vi "Main.vi"() -> ()   [LabVIEW 2017]
uses:
  mode_tab.ctl
  state_history.ctl
  <vilib>/Utility/miscctls.llb/LVPointTypeDef.ctl
  <vilib>/Utility/error.llb/DialogType.ctl
  <instrlib>/Gantner Instruments/Ethernet/Gantner-Instruments HighSpeedPort.llb/e.gate Protocol Type.ctl
  global_variable_GAUGE_PANEL_ERROR.vi
  global_variable_STOP.vi
panel:
  out "State History":T1 {"Time Stamp" format="%<%I:%M:%S %p>T"}
  out "STATUS":string
  in  "pause button":bool
  in  "return button":bool
  in  "Mode Tab":T2
  in  "DAQ IP Address":string="192.168.1.28"
  in  "ignore limit switch feedback":bool
  in  "RUN":bool
  in  "debug - run a state":string
  in  "stop program":bool
  in  "set default state":bool
  in  "demo mode":bool
  in  "proceed button":bool
  out "LAST ERROR":errorcluster
  in  "error in (no error)":errorcluster
  out "error out":errorcluster
  # "VIRTUAL CONTROL BOX is still in for loop when program stops connection"
  # "make it easier to add tabs to program"
  # "TAB CONTROL IS NOT RESIZING"
  # "actuation error causes a paused execution (FIXED BY SETTING \"ALLOW DEBUGGING\" TO BE FALSE in vi properties)"
  # "Debug Zone"
  # "The buttons below are now enabled"
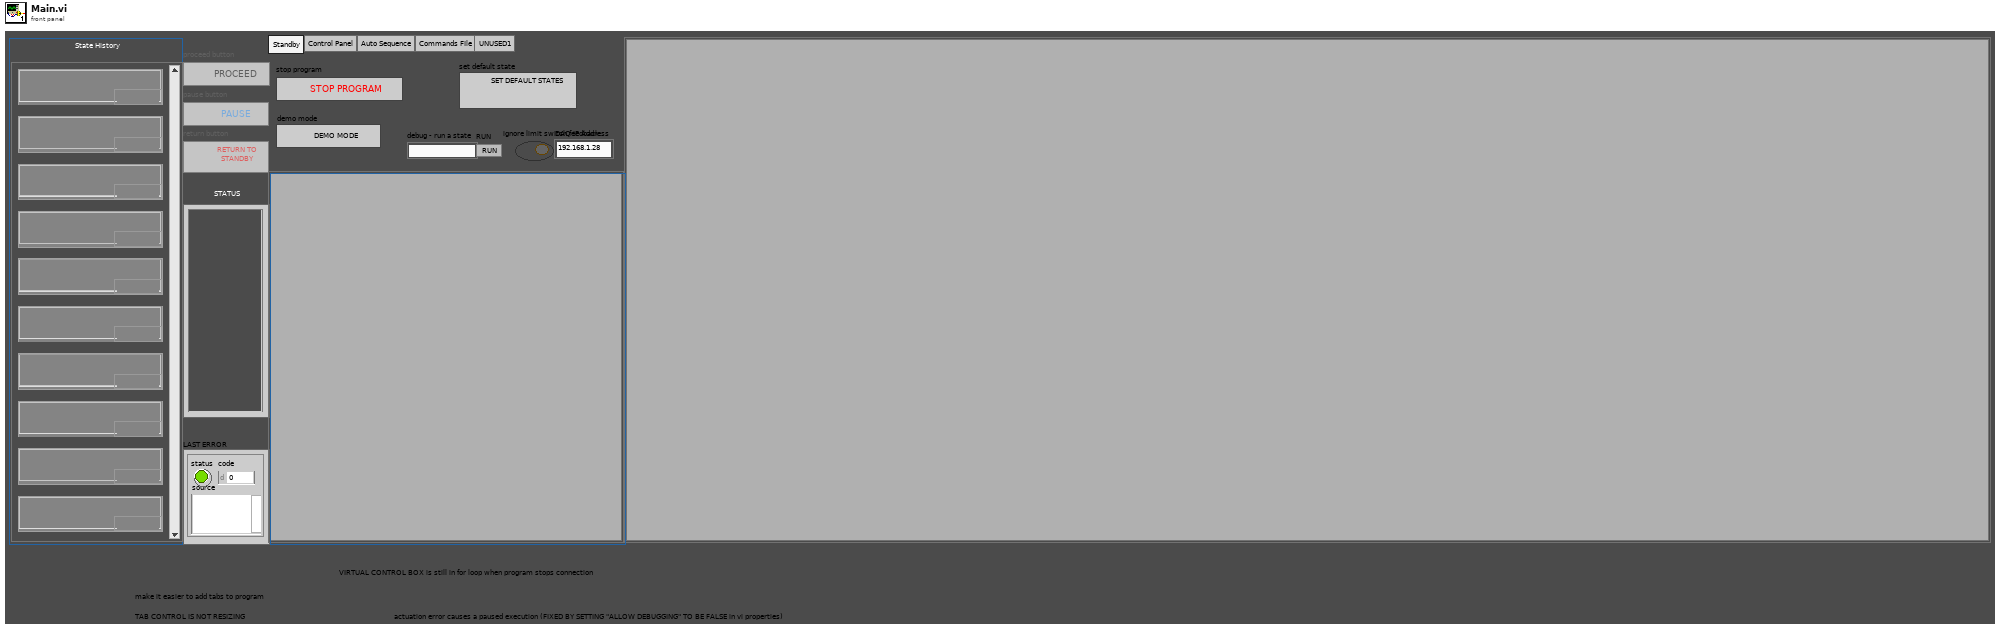
[diagram p1: front panel]
types:
  T1 = typedef "state_history.ctl" = cluster{"String":string, "Time Stamp":timestamp}[]
  T2 = typedef "mode_tab.ctl" = enum32{"Standby", "Control Panel", "Auto Sequence", "Commands FIle", "UNUSED1"}
  T3 = typedef "LVPointTypeDef.ctl" = cluster{"Horizontal":i16, "Vertical":i16}
  T4 = cluster{"name (unnamed)":string, "seconds since 1Jan1904":timestamp}
  T5 = cluster{"name (unnamed)":string, "current time":timestamp}[]
  T6 = enum32{"Invalid", "Standard", "Closed", "Hidden", "Minimized", "Maximized"}
  T7 = enum32{"invalid app kind", "Development System", "Run Time System", "Student Edition", "Embedded LabVIEW", "Evaluation", "Custom"}
  T8 = enum8{"Enabled", "Disabled", "Disabled and Grayed Out"}
  T9 = enum32{"Page Enabled", "Page Disabled", "Page Disabled & Grayed"}
  T10 = enum16{"open/close=1/0", "open/close=0/1", "on/off=1/0", "on/off=0/1"}
  T11 = enum16{"open/close=1/0", "open/close=0/1", "on/off=1/0", "on/off=0/1", "logger_progress"}
  T12 = cluster{"Core":cluster{"Current VI Reference":refnum<vi>, "Close Panel on Exit?":bool}, "time1":dbl, "timeout":dbl, "digital logic":enum16{"open/close=1/0", "open/close=0/1", "on/off=1/0", "on/off=0/1", "logger_progress"}, "channel name":string, "winch parameter":dbl, "proceed button":refnum<vi>, "Mode Tab":refnum<vi>, "mode":enum16{"online", "demo", "compile"}}
  T13 = typedef "DialogType.ctl" = u16
  T14 = cluster{"Current VI Reference":refnum<vi>, "Close Panel on Exit?":bool}
  T15 = typedef "e.gate Protocol Type.ctl" = enum16{"ASCII", "HighspeedPort Online", "HighspeedPort Buffer (giutility.DLL) ", "PostProcessBuffer (giutility.DLL)"}
  T16 = typedef "e.gate Configuration.ctl" = cluster{"connection ID":refnum<k5>, "IPAddress":string, "BufferIndex":i32, "StateMessage":string, "StateCode":i8, "HeaderSize":i32, "BufferSize":i32, "IsBigEndian":i32, "Version":i32, "ChannelCount":i32, "FrameLength":i32, "StartTime":dbl, "dActTimeToSecondFactor":dbl, "StartTimeToDayFactor":dbl, "BufferFillRate":dbl, "SampleRate":dbl, "ChannelData":T17[], "DecodeTimeFormat":string, "SummaryPath":string, "WithCheckSum":i32, "dActTimeDataType":T18, "MaxWriteCount":i32, "MaxReadCount":i32, "TempOffsetRead":i32, "TempLengthRead":i32, "Protocol":T15, "IsSupported":i32, "InputAccessList":i32[], "OutputAccessList":i32[], "DataSource":enum16{"CircleBuffer", "test.con Logger", "test.con Archive"}, "Modules":T19[], "DLL-Handle":T20}
  T17 = typedef "e.gate Channel Data.ctl" = cluster{"VariableName":string, "DataDirection":string, "DataType":string, "DataTypeIndex":T18, "Precision":i16, "FieldLengtht":i16, "ByteCount":i32, "Format":string, "Unit":string, "InputAccessOffset":i32, "OutputAccessOffset":i16, "InputAccessIndex":i16, "OutputAccessIndex":i16, "VarType":string}
  T18 = typedef "e.gate Data Type.ctl" = enum16{"NO", "BOOL", "SINT8", "USINT8", "SINT16", "USINT16", "SINT32", "USINT32", "FLOAT", "SET8", "SET16", "SET32", "DOUBLE", "SINT64", "USINT64", "SET64"}
  T19 = typedef "e.gate Module  Data.ctl" = cluster{"Type":string, "Location":string, "VariablesCount":i16, "UartIndex":i16, "Address":i16, "SystemOffset":i16}
  T20 = typedef "e.gateHSP_DLLhandle.ctl" = cluster{"clientInstance":i32, "connectionInstance":i32, "Is32Bit":bool, "DLL Path":path}
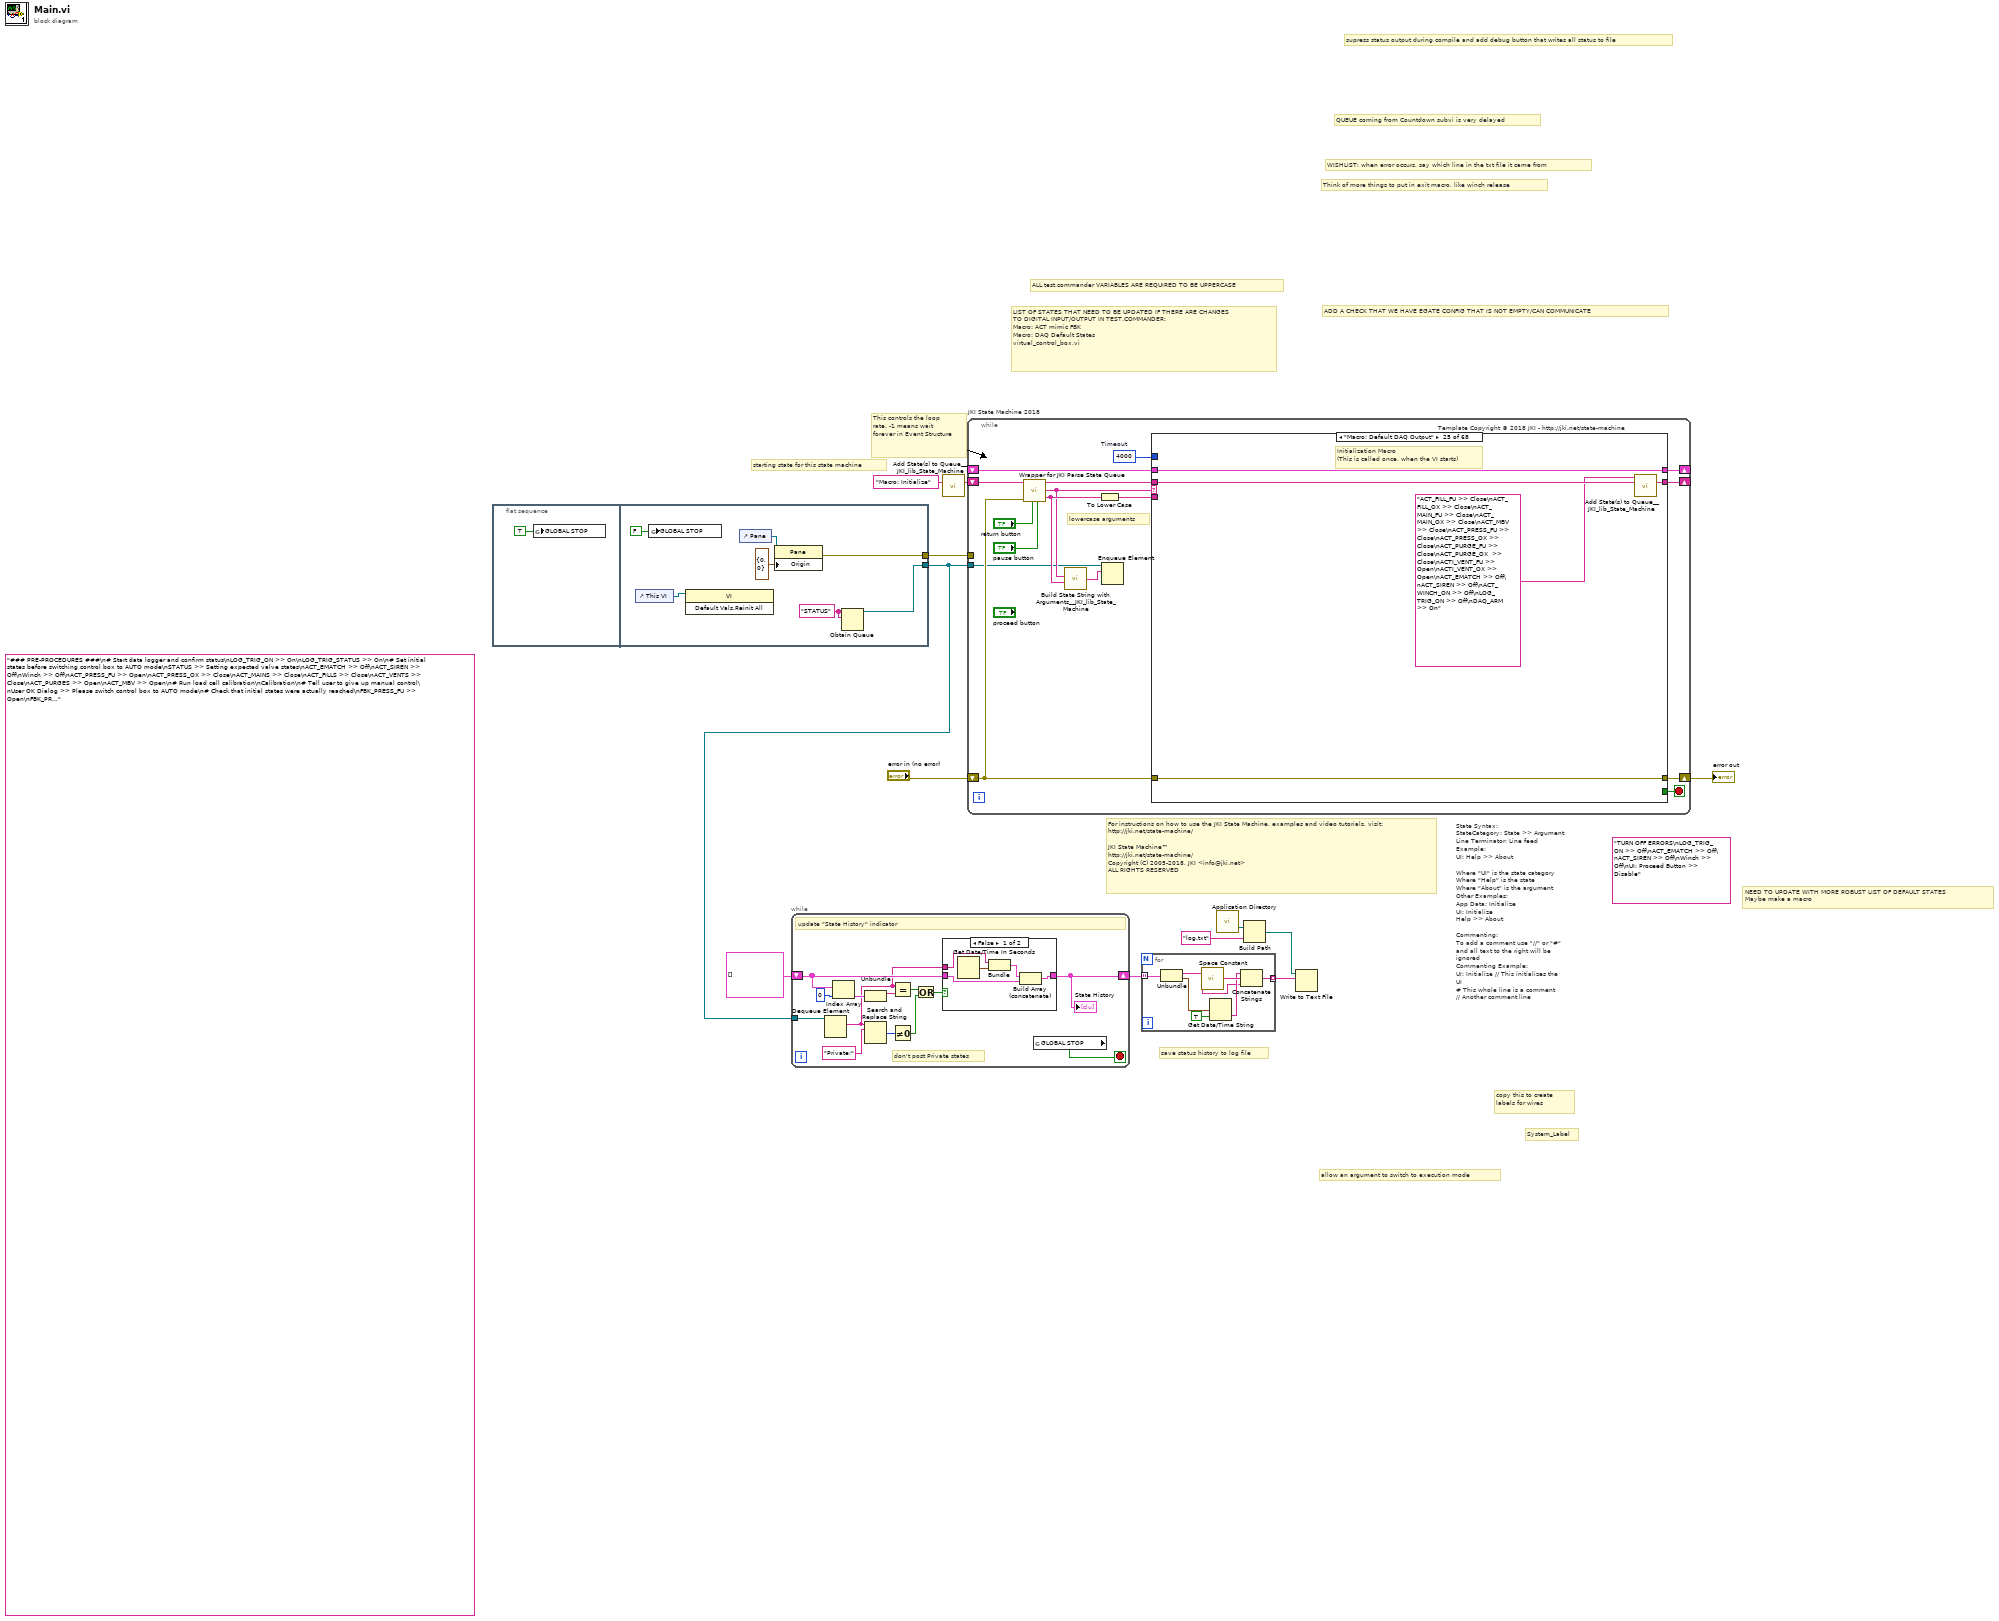
[diagram p0: block diagram]
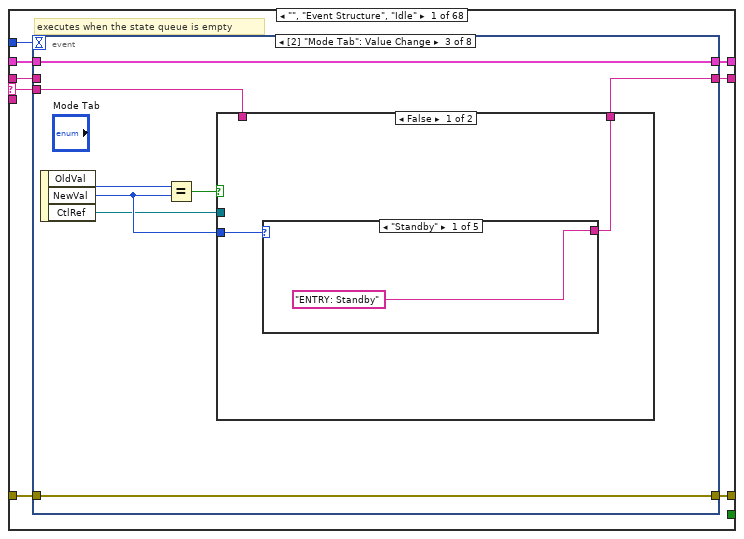
[diagram p3: hidden frame]
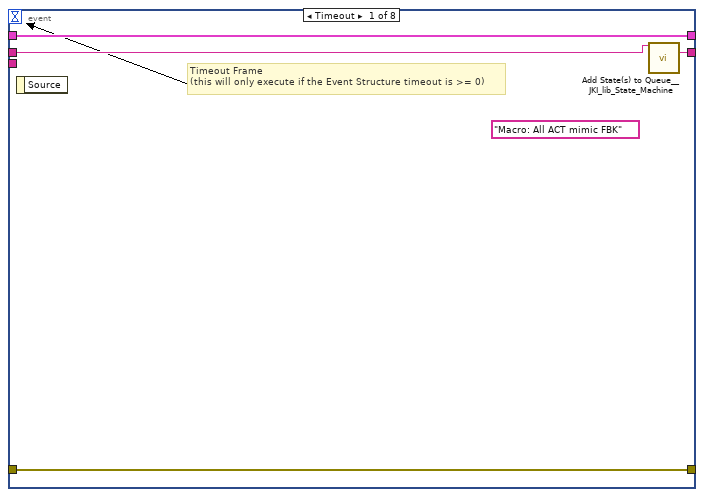
[diagram p4: hidden frame]
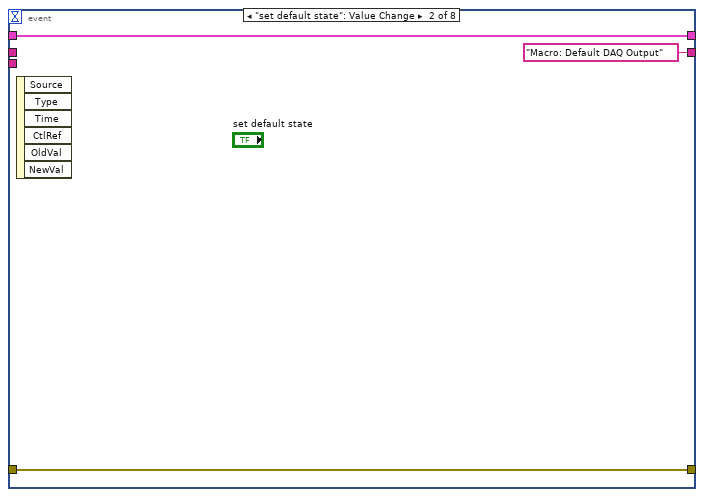
[diagram p5: hidden frame]
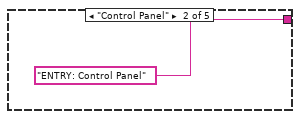
[diagram p6: hidden frame]
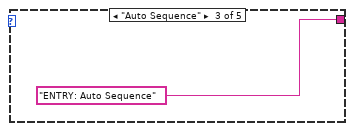
[diagram p7: hidden frame]
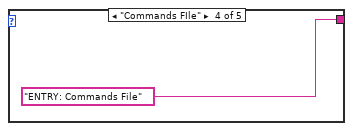
[diagram p8: hidden frame]
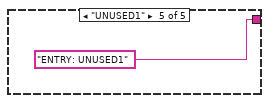
[diagram p9: hidden frame]
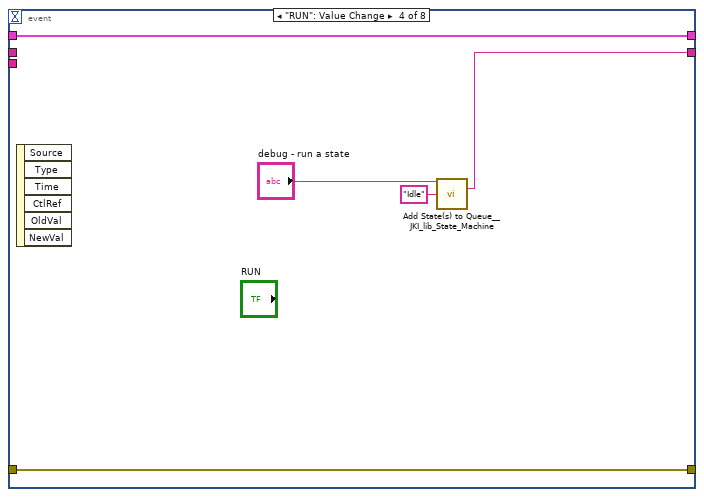
[diagram p11: hidden frame]
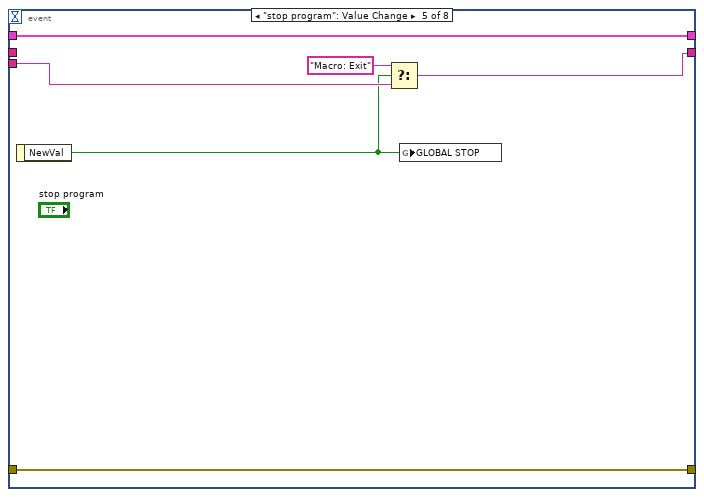
[diagram p12: hidden frame]
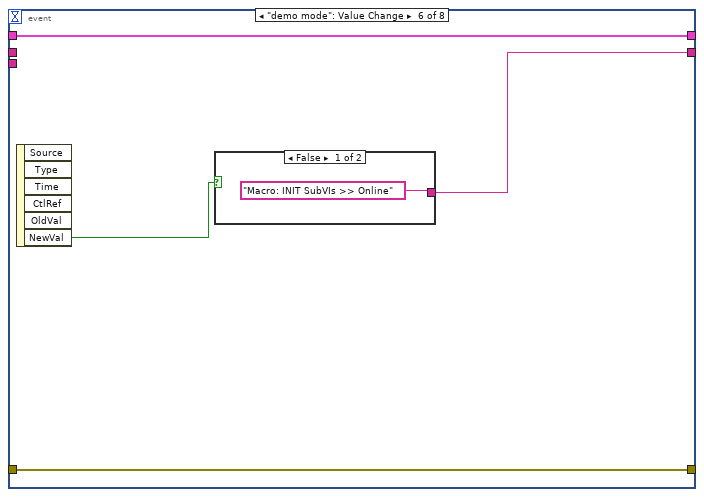
[diagram p13: hidden frame]
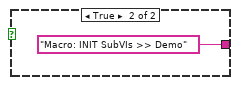
[diagram p14: hidden frame]
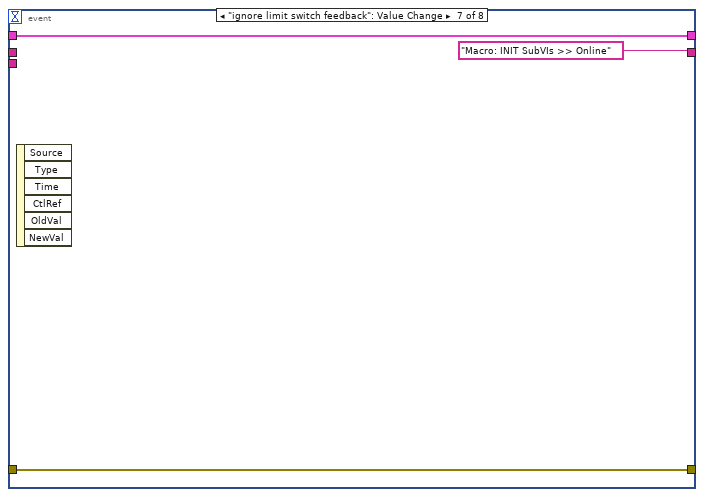
[diagram p15: hidden frame]
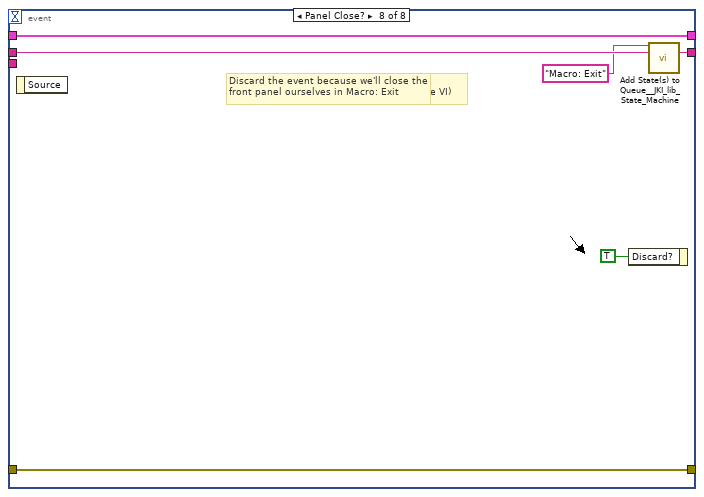
[diagram p16: hidden frame]
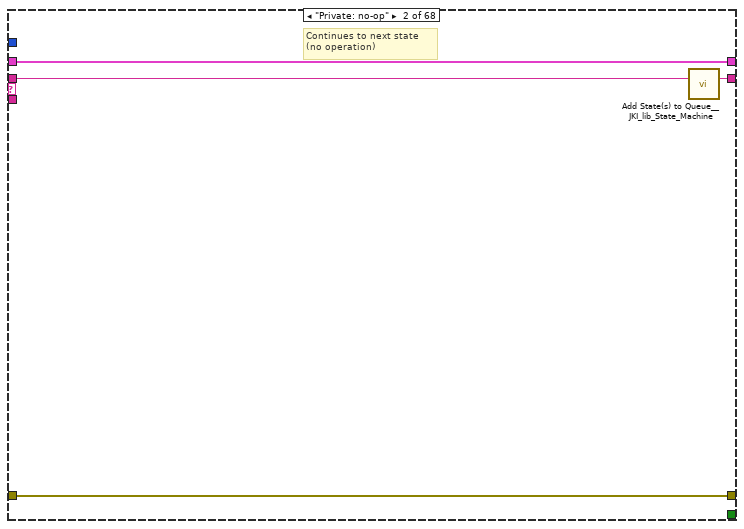
[diagram p17: hidden frame]
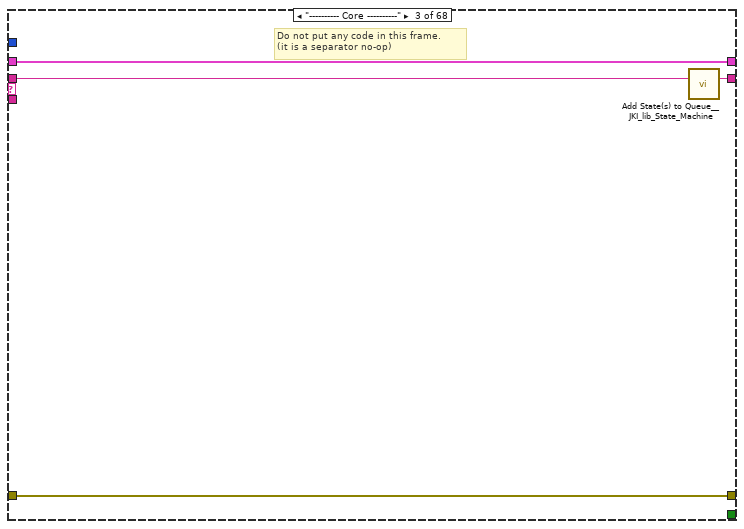
[diagram p18: hidden frame]
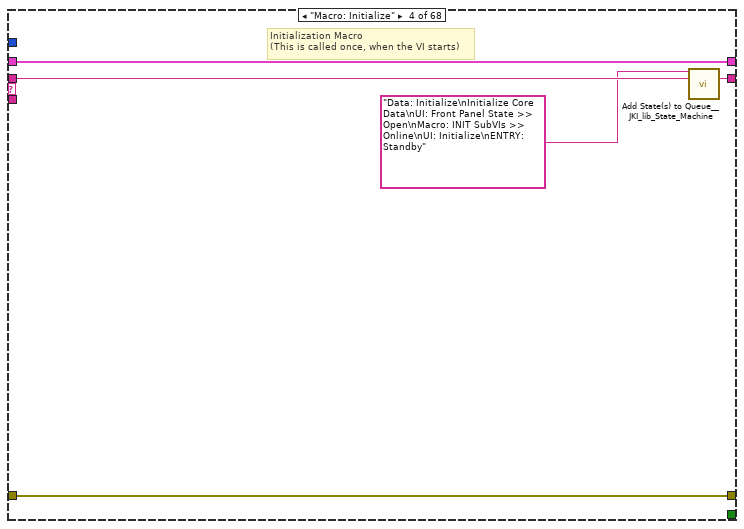
[diagram p19: hidden frame]
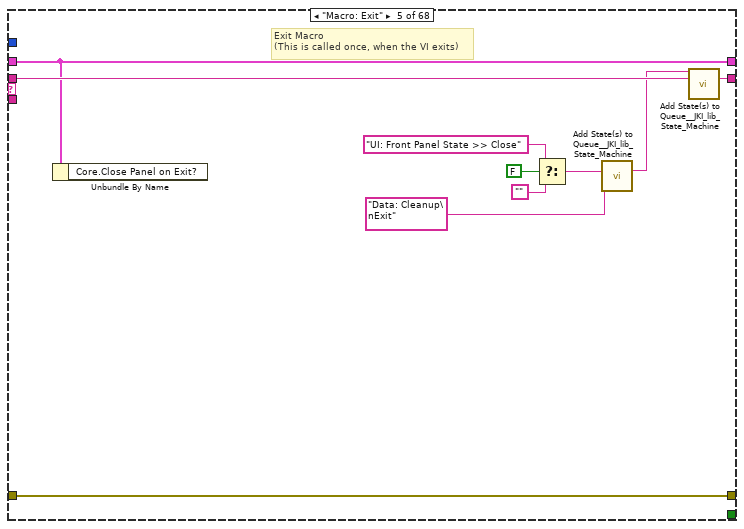
[diagram p20: hidden frame]
diagram:
  (unwired) "TURN OFF ERRORS\nLOG_TRIG_ON >> Off\nACT_EMATCH >> Off\nACT_SIREN >> Off\nWinch >> Off\nUI: Proceed Button >> Disable" ("State(s) in Front (\"\")")
  (unwired) "### PRE-PROCEDURES ###\n# Start data logger and confirm status\nLOG_TRIG_ON >> On\nLOG_TRIG_STATUS >> On\n# Set initial states before switching control box to AUTO mode\nSTATUS >> Setting expected valve states\nACT_EMATCH >> Off\nACT_SIREN >> Off\nWinch >> Off\nACT_PRESS_FU >> Open\nACT_PRESS_OX >> Close\nACT_MAINS >> Close\nACT_FILLS >> Close\nACT_VENTS >> Close\nACT_PURGES >> Open\nACT_MBV >> Open\n# Run load cell calibration\nCalibration\n# Tell user to give up manual control\nUser OK Dialog >> Please switch control box to AUTO mode\n# Check that initial states were actually reached\nFBK_PRESS_FU >> Open\nFBK_PRESS_OX >> Close\nFBK_MAIN_FU >> Close\nFBK_MAIN_OX >> Close\nFBK_FILL_FU >> Close\nFBK_FILL_OX >> Close\nFBK_VENT_FU >> Close\nFBK_VENT_OX >> Close\nFBK_PURGE_FU >> Open\nFBK_PURGE_OX >> Open\nFBK_MBV_OPENED >> Open\n### PROCEDURES ###\n# Begin OX Tank pressurization\nACT_PRESS_OX >> Open\nFBK_PRESS_OX >> Open\nWait for OX Tank Pressure >> 1000 //THE PRESSURE (PSI) THAT THE OX TANK SHOULD REACH\n# Begin countdown procedures\nACT_PURGE_FU >> Close\nACT_PURGE_OX >> Close\nFBK_PURGE_FU >> Close\nFBK_PURGE_OX >> Close\nACT_SIREN >> On\nStart Countdown >> 3 //NUMBER OF SECONDS BETWEEN TURNING ON IGNITION AND OPENING MAIN VALVES\nACT_EMATCH >> On\nACT_SIREN >> Off\nWait >> 3 //NUMBER OF SECONDS BETWEEN TURNING ON IGNITION AND OPENING MAIN VALVES (same as above)\nACT_MAIN_OX >> Open\nWait >> 0.25 //NUMBER OF SECONDS BETWEEN OPENING OX MAIN VALVE AND FU MAIN VALVE\nACT_MAIN_FU >> Open\nFBK_MAIN_OX >> Open\nFBK_MAIN_FU >> Open\n### FIRE ###\nWait >> 0.5 //NUMBER OF SECONDS AFTER THE START OF BURN TO TURN OFF IGNITION (counts towards total burn time)\nACT_EMATCH >> Off\nWait >> 1.5 //NUMBER OF SECONDS AFTER IGNITION TURNS OFF TO OPEN THE PURGES (counts towards total burn time)\nACT_PURGE_FU >> Open\nACT_PURGE_OX >> Open\nWait >> 9 //NUMBER OF SECONDS AFTER PURGES OPEN TO CONTINUE THE BURN (counts towards total burn time)\n### GRACEFUL END ###\nACT_MAIN_OX >> Close\nACT_MAIN_FU >> Close\nFBK_MAIN_OX >> Close\nFBK_MAIN_FU >> Close\nWait >> 4 //NUMBER OF SECONDS TO KEEP PURGES OPEN AFTER MAIN VALVES CLOSED\nACT_PURGE_FU >> Close\nACT_PURGE_OX >> Close\n\n///// probably put the following before purges close ////////\nACT_VENT_FU >> Open\nACT_VENT_OX >> Open\nACT_PRESS_FU >> Close\nACT_PRESS_OX >> Close\nACT_MBV >> Close\n//////  ///////\n\nFBK_MBV_CLOSED >> Close\n\n//////// still need to do this?? ////////\nACT_PRESS_FU >> Open\nFBK_PRESS_OX >> Open\nWait >> 2\nACT_PRESS_FU >> Close\nACT_PRESS_OX >> Close\n//////  ///////\n\n### FINISH ###\nLOG_TRIG_ON >> Off\nWait >> 30\n###Ask to run cleanup?"
  # "save status history to log file"
  # "ALL test.commander VARIABLES ARE REQUIRED TO BE UPPERCASE"
  # "LIST OF STATES THAT NEED TO BE UPDATED IF THERE ARE CHANGES\nTO DIGITAL INPUT/OUTPUT IN TEST.COMMANDER:\nMacro: ACT mimic FBK\nMacro: DAQ Default States\nvirtual_control_box.vi"
  # "allow an argument to switch to execution mode"
  # "supress status output during compile and add debug button that writes all status to file"
  # "NEED TO UPDATE WITH MORE ROBUST LIST OF DEFAULT STATES\nMaybe make a macro"
  # "QUEUE coming from Countdown subvi is very delayed"
  # "WISHLIST: when error occurs, say which line in the txt file it came from"
  # "starting state for this state machine"
  # "Think of more things to put in exit macro, like winch release"
  # "ADD A CHECK THAT WE HAVE EGATE CONFIG THAT IS NOT EMPTY/CAN COMMUNICATE"
  # "For instructions on how to use the JKI State Machine, examples and video tutorials, visit:\nhttp://jki.net/state-machine/\n\nJKI State Machine™\nhttp://jki.net/state-machine/\nCopyright (C) 2005-2018, JKI <info@jki.net>\nALL RIGHTS RESERVED"
  # "State Syntax:\nStateCategory: State >> Argument\nLine Terminator: Line feed\nExample:\nUI: Help >> About\n\nWhere \"UI\" is the state category\nWhere \"Help\" is the state\nWhere \"About\" is the argument\nOther Examples:\nApp Data: Initialize\nUI: Initialize\nHelp >> About\n\nCommenting:\nTo add a comment use \"//\" or \"#\" and all text to the right will be ignored\nCommenting Example:\nUI: Initialize // This initializes the UI\n# This whole line is a comment\n// Another comment line"
  # "copy this to create labels for wires"
  # "This controls the loop rate. -1 means wait forever in Event Structure"
  # "System_Label"
  n1 = flat-sequence {
    tunnel: [w17] -> w6
    tunnel: [w14] -> w4
    frame #0 {
      n2 = global write "global_variable_STOP.vi" "GLOBAL STOP"(TRUE ("GLOBAL STOP")) -> ()
    }
    frame #1 {
      w15 = "STATUS" ("name (unnamed)")
      n3 = control-ref of="This VI"() -> (w20:refnum<vi>)
      n4 = global write "global_variable_STOP.vi" "GLOBAL STOP"(FALSE ("GLOBAL STOP")) -> ()
      n5 = invoke class="VI" method="Default Vals.Reinit All"(reference=w20) -> ()  [unwired: 2 in, 3 out]
      n6 = control-ref of="Pane"() -> (w18:refnum<vi>)
      n7 = property class="Pane"(reference=w18, "Origin"=T3 {"Horizontal"=0, "Vertical"=0}) -> (error out=w17:errorcluster)  [unwired: 1 in, 1 out]
      n8 = Obtain Queue(name (unnamed)=w15, element data type=w15) -> (queue out=w14:refnum<queue>)  [unwired: 3 in, 2 out]
    }
  }
  n9 = while {
    shift-right: [w21] -> w9
    shift-left: cluster{string, "current time":timestamp}[] [] -> [w31]
    tunnel: w4 -> [w22]
    stop <- w23 stop-if-true
    # "don't post Private states"
    # "update \"State History\" indicator"
    n10 = Dequeue Element(queue=w22) -> (element=w27:string)  [unwired: 2 in, 3 out]
    n11 = Index Array(array=w31, index=0) -> (element=w32:cluster{string, "current time":timestamp})
    n12 = Unbundle(w32) -> (w30:string)  [unwired: 1 out]
    n13 = Search and Replace String(input string=w27, search string="Private:") -> (number of replacements=w26:i32)  [unwired: 6 in, 3 out]
    n14 = Equal?(x=w27, y=w30) -> (x = y?=w29:bool)
    n15 = Not Equal To 0?(x=w26) -> (x != 0?=w24:bool)
    n16 = Or(x=w29, y=w24) -> (x .or. y?=w25:bool)
    n17 = case shown="False" w25 {
      tunnel: [w38 w39] -> w21
      tunnel: w27 -> [w37 _]
      tunnel: w31 -> [w35 w39]
      frame False {
        n18 = Get Date/Time In Seconds() -> (seconds since 1Jan1904=w34:timestamp)
        n19 = Bundle("name (unnamed)"=w37, "seconds since 1Jan1904"=w34) -> (w36:T4)  [unwired: 1 in]
        n20 = Build Array (concatenate)(w36, w35) -> (w38:T5)
      }
      frame True {
      }
    }
    "State History" <- w21
    n21 = global read "global_variable_STOP.vi" "GLOBAL STOP"() -> (w23:bool)
  }
  n22 = call <vilib>:"Add State(s) to Queue__JKI_lib_State_Machine.vi"("State(s) in (\"\")"="Macro: Initialize") -> ("States Out"=w12:string)  [unwired: 14 in]
  n23 = while "JKI State Machine 2018" {
    shift-right: [w52] -> _
    shift-left: _ -> [w51]
    shift-right: [w55] -> w5
    shift-left: "error in (no error)" -> [w47]
    shift-right: [w54] -> _
    shift-left: w12 -> [w46]
    tunnel: w6 -> [_]
    tunnel: w4 -> [w41]
    stop <- w53 stop-if-true
    w50 = 4000  # Timeout
    # "lowercase arguments"
    # "Template Copyright © 2018 JKI - http://jki.net/state-machine"
    n24 = call "Wrapper for JKI Parse State Queue.vi"("pause execution"="pause button", "cancel execution"="return button", "error in (no error)"=w47, "State Queue"=w46) -> ("Arguments"=w43:string, "Current State"=w42:string, "Remaining States"=w48:string)  [unwired: 5 in]
    n25 = call <vilib>:"Build State String with Arguments__JKI_lib_State_Machine.vi"("Arguments (\"\")"=w43, "State"=w42) -> ("State with Arguments"=w40:string)  [unwired: 4 in]
    n26 = To Lower Case(string=w43) -> (all lower case string=w49:string)
    n27 = Enqueue Element(queue=w41, element=w40) -> ()  [unwired: 2 in, 3 out]
    n28 = case shown="\"Macro: Default DAQ Output\"" w42 {
      selector: w42 -> [w56 _ _ _ _ w136 _ _ _ _ _ _ _ _ _ _ _ _ _ _ _ _ _ _ _ _ _ _ _ _ _ _ _ _ _ _ _ _ w690 w732 w762 _ _ _ _ w837 w849 _ w941 w982 _ _ _ _ _ w1058 w1068 w1078 _ w1114 w1186 w1203 w1220 w1237 _ _ _ _]
      tunnel: w48 -> [w63 w116 w120 w125 w135 w140 w159 w166 w222 w226 w239 w245 w249 w254 w260 w271 w345 w368 w378 w391 w404 w414 w424 w430 w435 w437 w443 w459 w477 w492 w497 w513 w519 w525 w538 w625 w627 w634 w675 w734 w763 w768 w790 w795 w801 w834 w846 w885 w904 w945 w987 w1002 w1006 w1010 w1011 w1067 w1077 w1087 w1091 w1119 w1188 w1205 w1222 w1239 w1250 w1256 w1261 w1264]
      tunnel: w49 -> [_ _ _ _ _ _ _ _ _ _ _ _ _ _ w255 w265 w343 w362 w372 w387 w401 w409 _ _ _ _ _ w448 _ _ _ w512 _ _ w553 _ _ w646 w689 w725 w748 w767 _ w791 w803 w836 w848 w870 w916 w963 w989 _ _ _ w1015 w1063 w1073 w1083 _ w1111 w1183 w1200 w1217 w1234 _ _ _ w1263]
      tunnel: w51 -> [w61 w113 w117 w122 w132 w138 w152 w163 w220 w223 _ w240 w246 w250 w258 w267 w340 w365 w375 w385 w400 w411 w421 w425 w432 w439 w445 w457 w481 w494 w509 w514 w521 w536 w552 w622 w628 w633 w673 w735 w747 w765 w787 w792 w806 w825 w844 w883 w932 w976 w986 w999 w1003 w1007 w1017 w1061 w1071 w1081 w1088 w1105 w1193 w1210 w1227 w1244 w1247 w1251 w1258 w1275]
      tunnel: [w60 w114 w118 w123 w133 w142 w156 w165 w219 w224 w236 w241 w247 w252 w256 w268 w341 w366 w376 w383 w402 w412 w422 w428 w433 w440 w446 w455 w478 w495 w498 w511 w522 w526 w540 w623 w629 w642 w682 w730 w759 w769 w788 w793 w810 w833 w845 w886 w939 w980 w988 w1000 w1004 w1008 w1019 w1065 w1075 w1085 w1089 w1116 w1194 w1211 w1228 w1245 w1248 w1254 w1259 w1266] -> w55
      tunnel: w47 -> [w59 w114 w118 w123 w133 w141 w156 w167 w219 w224 w236 w242 w247 w252 w257 w269 w342 w366 w376 w384 w402 w412 w422 w428 w433 w440 w446 w456 w478 w495 w499 w511 w522 w527 w550 w623 w629 w644 w687 w731 w761 w770 w788 w793 w809 w833 w845 w860 w939 w980 w988 w1000 w1004 w1008 w1018 w1065 w1075 w1085 w1089 w1110 w1194 w1211 w1228 w1245 w1248 w1254 w1259 w1267]
      tunnel: [w62 w115 w119 w124 w134 w139 w158 w170 w221 w225 w238 w244 w248 w253 w259 w270 w344 w367 w377 w390 w403 w413 w423 w429 w434 w441 w447 w458 w482 w496 w510 w515 w523 w537 w559 w624 w630 w657 w696 w736 w764 w771 w789 w794 w813 w840 w852 w887 w942 w983 w990 w1001 w1005 w1009 w1020 w1066 w1076 w1086 w1090 w1118 w1195 w1212 w1229 w1246 w1249 w1255 w1260 w1276] -> w54
      tunnel: [_ _ _ _ _ _ _ w164 TRUE _ _ _ _ _ _ _ _ _ _ _ _ _ _ _ _ _ _ _ _ _ _ _ _ _ _ _ _ _ _ _ _ _ _ _ _ _ _ _ _ _ _ _ _ _ _ _ _ _ _ _ _ _ _ _ _ _ _ _] -> w53
      tunnel: [w58 w113 w117 w122 w132 w138 w157 w163 w220 w223 w237 w240 w246 w250 w258 w267 w340 w365 w375 w385 w400 w411 w421 w425 w432 w439 w445 w457 w481 w494 w509 w514 w521 w536 w551 w622 w628 w640 w672 w735 w747 w765 w787 w792 w804 w825 w844 w881 w932 w976 w986 w999 w1003 w1007 w1017 w1060 w1070 w1080 w1088 w1105 w1192 w1209 w1226 w1243 w1247 w1251 w1258 w1275] -> w52
      tunnel: w50 -> [w57 _ _ _ _ _ _ _ _ _ _ _ _ _ _ _ _ _ _ _ _ _ _ _ _ _ _ _ _ _ _ _ _ _ _ _ _ _ _ _ _ _ _ _ _ _ _ _ _ _ _ _ _ _ _ _ _ _ _ _ _ _ _ _ _ _ _ _]
      frame "", "Event Structure", "Idle" {
        # "executes when the state queue is empty"
        n29 = event shown="[2] \"Mode Tab\": Value Change" {
          selector: _ -> [_ _ _ _ _ _ _ _]
          dyn-events: _ -> [_ _ _ _ _ _ _ _]
          timeout: w57 -> [_ _ _ _ _ _ _ _]
          tunnel: w63 -> [w64 _ _ _ _ _ _ w112]
          tunnel: [w67 "Macro: Default DAQ Output" ("States Out") w73 w87 w95 w101 "Macro: INIT SubVIs >> Online" ("States Out") w111] -> w62
          tunnel: w61 -> [w65 w68 w76 w91 w94 w98 w104 w109]
          tunnel: [w66 w69 w75 w90 w93 w99 w105 w110] -> w60
          tunnel: w59 -> [w66 w69 w75 w90 w93 w99 w105 w110]
          tunnel: [w65 w68 w76 w91 w94 w98 w104 w109] -> w58
          tunnel: w56 -> [_ _ w72 _ w97 _ _ _]
          event Timeout {
            (unwired) "Macro: All ACT mimic FBK" ("State(s) in Front (\"\")")
            # "Timeout Frame\n(this will only execute if the Event Structure timeout is >= 0)"
            n30 = event-data() -> ()  [unwired: 1 in, 1 out]
            n31 = call <vilib>:"Add State(s) to Queue__JKI_lib_State_Machine.vi"("State(s) in Front (\"\")"=w64) -> ("States Out"=w67:string)  [unwired: 14 in]
          }
          event "set default state": Value Change {
            n32 = event-data() -> ()  [unwired: 1 in, 6 out]
          }
          event Value Change {
            n33 = event-data() -> ("OldVal"=w77:T2, "NewVal"=w74:T2, "CtlRef"=w71:refnum<vi>)  [unwired: 1 in]
            n34 = Equal?(x=w77, y=w74) -> (x = y?=w78:bool)
            n35 = case shown="False" w78 {
              tunnel: [w79 w86] -> w73
              tunnel: w74 -> [w80 _]
              tunnel: w72 -> [_ w86]
              tunnel: w71 -> [_ _]
              frame False {
                n36 = case shown="\"Standby\"" w80 {
                  tunnel: ["ENTRY: Standby" "ENTRY: Control Panel" "ENTRY: Auto Sequence" ("string") "ENTRY: Commands File" "ENTRY: UNUSED1"] -> w79
                  frame "Standby" {
                  }
                  frame "Control Panel" {
                  }
                  frame "Auto Sequence" {
                  }
                  frame "Commands FIle" {
                  }
                  frame "UNUSED1" {
                  }
                }
              }
              frame True {
              }
            }
          }
          event "RUN": Value Change {
            n37 = event-data() -> ()  [unwired: 1 in, 6 out]
            n38 = call <vilib>:"Add State(s) to Queue__JKI_lib_State_Machine.vi"("State(s) in Front (\"\")"="debug - run a state", "State(s) at Back (\"\")"="Idle" ("State(s) at Back (\"\")")) -> ("States Out"=w87:string)  [unwired: 13 in]
          }
          event "stop program": Value Change {
            n39 = event-data() -> ("NewVal"=w92:bool)  [unwired: 1 in]
            n40 = Select(t="Macro: Exit", s=w92, f=w97) -> (s? t:f=w95:string)
            n41 = global write "global_variable_STOP.vi" "GLOBAL STOP"(w92) -> ()
          }
          event "demo mode": Value Change {
            n42 = event-data() -> ("NewVal"=w100:bool)  [unwired: 1 in, 5 out]
            n43 = case shown="False" w100 {
              tunnel: ["Macro: INIT SubVIs >> Online" ("States Out") "Macro: INIT SubVIs >> Demo" ("States Out")] -> w101
              frame False {
              }
              frame True {
              }
            }
          }
          event "ignore limit switch feedback": Value Change {
            n44 = event-data() -> ()  [unwired: 1 in, 6 out]
          }
          event Panel Close? {
            # "Discard the event because we'll close the front panel ourselves in Macro: Exit"
            # "Close Panel button (pressed) Event\n(this executes Macro: Exit to terminate the VI)"
            n45 = event-data() -> ()  [unwired: 1 in, 1 out]
            n46 = event-data("Discard?"=TRUE) -> ()  [unwired: 1 in, 1 out]
            n47 = call <vilib>:"Add State(s) to Queue__JKI_lib_State_Machine.vi"("State(s) in Front (\"\")"="Macro: Exit", "State(s) in (\"\")"=w112) -> ("States Out"=w111:string)  [unwired: 13 in]
          }
        }
      }
      frame "Private: no-op" {
        # "Continues to next state\n(no operation)"
        n48 = call <vilib>:"Add State(s) to Queue__JKI_lib_State_Machine.vi"("State(s) in (\"\")"=w116) -> ("States Out"=w115:string)  [unwired: 14 in]
      }
      frame "---------- Core ----------" {
        # "Do not put any code in this frame.\n(it is a separator no-op)"
        n49 = call <vilib>:"Add State(s) to Queue__JKI_lib_State_Machine.vi"("State(s) in (\"\")"=w120) -> ("States Out"=w119:string)  [unwired: 14 in]
      }
      frame "Macro: Initialize" {
        # "Initialization Macro\n(This is called once, when the VI starts)"
        n50 = call <vilib>:"Add State(s) to Queue__JKI_lib_State_Machine.vi"("State(s) in Front (\"\")"="Data: Initialize\nInitialize Core Data\nUI: Front Panel State >> Open\nMacro: INIT SubVIs >> Online\nUI: Initialize\nENTRY: Standby", "State(s) in (\"\")"=w125) -> ("States Out"=w124:string)  [unwired: 13 in]
      }
      frame "Macro: Exit" {
        # "Exit Macro\n(This is called once, when the VI exits)"
        n51 = Unbundle By Name(w132) -> ()  [unwired: 1 out]
        n52 = Select(t="UI: Front Panel State >> Close", s=FALSE, f="") -> (s? t:f=w129:string)
        n53 = call <vilib>:"Add State(s) to Queue__JKI_lib_State_Machine.vi"("State(s) in (\"\")"=w129, "State(s) at Back (\"\")"="Data: Cleanup\nExit") -> ("States Out"=w127:string)  [unwired: 13 in]
        n54 = call <vilib>:"Add State(s) to Queue__JKI_lib_State_Machine.vi"("State(s) in Front (\"\")"=w127, "State(s) in (\"\")"=w135) -> ("States Out"=w134:string)  [unwired: 13 in]
      }
      frame Default {
        w145 = 42 items=["No error", "Argument error", "Memory is full", "Out of zone", "End of file", "File already open", "Generic file I/O error", "File not found", "File permission error", "Disk is full", "Duplicate path", "Too many files open", "System feature not enabled", "Resource file not found", "Cannot add resource", "Resource not found", "Image not found", "Image memory error", "Pen does not exist", "Config type invalid", "Config token not found", "Config parse error", "Config memory error", "Bad external code format", "Bad external code offset", "External code not present", "Null window", "Destroy window error", "Null menu", "Print aborted", "Bad print record", "Print driver error", "Windows error during printing", "Memory error during printing", "Print dialog error", "Generic print error", "Invalid device refnum", "Device not found", "Device parameter error", "Device unit error", "Cannot open device", "Device call aborted", "Generic error", "Cancelled by user", "Object ID too low", "Object ID too high", "Object not in heap", "Unknown heap", "Unknown object (invalid DefProc)", "Unknown object (DefProc not in table)", "Message out of range", "Invalid (null) method", "Unknown message", "Manager call not supported", "Bad address", "Network operation in progress", "Network operation timed out", "Connection is busy", "Network attribute not supported", "Network error", "Address in use", "System out of memory", "Connection aborted", "Connection refused", "Not connected", "Already connected", "Connection closed", "Initialization error (interapplication manager)", "Bad occurrence", "Wait on unbound occurrence handler", "Occurrence queue overflow", "Datalog type conflict", "Unused", "Unrecognized type (interapplication manager)", "Memory corrupt", "Failed to make temporary DLL", "Old CIN version", "Drag socket not found", "Failed to load drop-object", "Failed to register OLE object", "Failed to release OLE object", "Format specifier type mismatch", "Unknown format specifier", "Too few format specifiers", "Too many format specifiers", "Scan failed", "Newer CIN version", "Error converting to variant", "Runtime menu error", "Password tampered", "Variant attribute not found", "Incompatible variant data type", "Event data is not available", "Event Store is not present", "Occurrence is not found", "Event Queue is not created", "Event info is not available", "Refnum passed is NULL", "Error retrieving Class GUID", "Error retrieving CoClass GUID", "Error retrieving TypeLib GUID.", "Bad built application magic bytes.", "Specific driver is different from the specific driver associated with the Logical Name.", "There is no session opened to the class driver.", "Max Error", "MAX - Error with config objects", "MAX - Error loading configuration", "MAX - Group not supported"]
        # "Current State"
        # "Do not delete, rename, or modify this frame.\n(this is used to capture unhandled states and typos)"
        # "Handle mistyped state name (developer tool)"
        n55 = Format Into String(format string="Software Exception: Unhandled State \"%s\"." ("message"), error in=w141, w136) -> (resulting string=w144:string, error out=w143:errorcluster)  [unwired: 1 in]
        n56 = call <vilib>:"Error Cluster From Error Code.vi"("show call chain? (False)"=TRUE, "error in (no error)"=w143, "error message (\"\")"=w144, "error code (0)"=w145) -> ("error out"=w142:errorcluster)  [unwired: 5 in]
        n57 = call <vilib>:"Add State(s) to Queue__JKI_lib_State_Machine.vi"("State(s) in (\"\")"=w140) -> ("States Out"=w139:string)  [unwired: 14 in]
      }
      frame "Initialize Core Data" {
        # "Do not delete, rename, or modify this frame.\n(this is used to determine panel behavior on exit)"
        # "originally closed?"
        # "exe?"
        # "If panel starts closed or is an EXE, then close it when we exit"
        n58 = property class="VI"() -> ("FP.State"=w149:T6)  [unwired: 2 in, 2 out]
        n59 = property class="App"() -> ("App.Kind"=w155:T7)  [unwired: 2 in, 2 out]
        n60 = control-ref of="Current VI Reference"() -> (w150:refnum<vi>)
        n61 = Equal?(x=w149, y=T6."Standard" ("Front Panel Window:State")) -> (x = y?=w147:bool)
        n62 = Equal?(x=w155, y=T7."Run Time System" ("Application:Kind")) -> (x = y?=w153:bool)
        n63 = Or(x=w147, y=w153) -> (x .or. y?=w151:bool)
        n64 = Bundle By Name(cluster=w152, "Core.Current VI Reference"=w150, "Core.Close Panel on Exit?"=w151) -> (w157:T12)
        n65 = call <vilib>:"Add State(s) to Queue__JKI_lib_State_Machine.vi"("State(s) in (\"\")"=w159) -> ("States Out"=w158:string)  [unwired: 14 in]
      }
      frame "Error Handler" {
        # "Handle any errors here.\nYou can also output any states to clean-up after errors occur"
        n66 = Unbundle By Name(w167) -> ("code"=w161:i32, "source"=w169:string)
        n67 = Unbundle By Name(w163) -> ("mode"=w162:enum16{"online", "demo", "compile"})
        n68 = case shown="Default" w162 {
          tunnel: w169 -> [w177 w199]
          tunnel: [w176 w198] -> w168
          tunnel: w167 -> [w175 w197]
          tunnel: w166 -> [_ w196]
          tunnel: [w173 w195] -> w165
          tunnel: [w172 w194] -> w164
          tunnel: w161 -> [w171 w192]
          tunnel: [w174 w193] -> w160
          frame "compile" {
            # "In this mode if we get a generic error it's probably a bad state from\nAUTO_SEQUENCE_COMMANDS.txt"
            n69 = case shown="66" w171 {
              tunnel: w177 -> [w178 w188 _]
              tunnel: [w178 "Macro: INIT SubVIs >> Online\nENTRY: Standby" "Macro: INIT SubVIs >> Online\nENTRY: Standby"] -> w176
              tunnel: w175 -> [w180 w184 w190]
              tunnel: [w182 w184 w190] -> w174
              tunnel: [w181 w185 w189] -> w173
              tunnel: [w179 _ _] -> w172
              frame Default {
                w179 = TRUE ("GLOBAL STOP")
                w183 = T13 2 items=["no dialog", "OK message", "continue or stop message", "OK message + warnings", "continue/stop + warnings"] ("type of dialog (OK msg:1)")
                n70 = global write "global_variable_STOP.vi" "GLOBAL STOP"(w179) -> ()
                n71 = call <vilib>:"General Error Handler.vi"("type of dialog (OK msg:1)"=w183, "error in (no error)"=w180) -> ("error out"=w182:errorcluster)  [unwired: 9 in, 4 out]
                n72 = call <vilib>:"Clear Errors.vi"("error in (no error)"=w180) -> ("error out"=w181:errorcluster)  [unwired: 5 in, 1 out]
              }
              frame 42 {
                # "generic error, unhandled state"
                n73 = One Button Dialog(message=w188, button name ("OK")="Return to Standby" ("T button name (\"OK\")")) -> ()  [unwired: 1 out]
                n74 = call <vilib>:"Clear Errors.vi"("error in (no error)"=w184) -> ("error out"=w185:errorcluster)  [unwired: 5 in, 1 out]
              }
              frame 66 {
                # "lost qstation connection"
                n75 = call <vilib>:"Clear Errors.vi"("error in (no error)"=w190) -> ("error out"=w189:errorcluster)  [unwired: 5 in, 1 out]
              }
            }
          }
          frame Default {
            n76 = case shown="66" w192 {
              tunnel: w199 -> [_ w212 _]
              tunnel: [w204 w209 "Macro: INIT SubVIs >> Online\nENTRY: Standby"] -> w198
              tunnel: w197 -> [w202 w206 w215]
              tunnel: w196 -> [w204 w208 _]
              tunnel: [w203 w207 w217] -> w195
              tunnel: [w201 _ _] -> w194
              tunnel: [w200 w206 w215] -> w193
              frame Default {
                w201 = TRUE ("GLOBAL STOP")
                w205 = T13 2 items=["no dialog", "OK message", "continue or stop message", "OK message + warnings", "continue/stop + warnings"] ("type of dialog (OK msg:1)")
                n77 = global write "global_variable_STOP.vi" "GLOBAL STOP"(w201) -> ()
                n78 = call <vilib>:"General Error Handler.vi"("type of dialog (OK msg:1)"=w205, "error in (no error)"=w202) -> ("error out"=w200:errorcluster)  [unwired: 9 in, 4 out]
                n79 = call <vilib>:"Clear Errors.vi"("error in (no error)"=w202) -> ("error out"=w203:errorcluster)  [unwired: 5 in, 1 out]
              }
              frame 108 {
                n80 = call <vilib>:"Clear Errors.vi"("error in (no error)"=w206) -> ("error out"=w207:errorcluster)  [unwired: 5 in, 1 out]
                n81 = Two Button Dialog(message=w212, 1:"Proceed Anyway (NOT RECOMMENDED)" ("F button name (\"Cancel\")"), 2:"Return to Standby" ("T button name (\"OK\")")) -> (T button?=w210:bool)
                n82 = Select(t="ENTRY: Standby", s=w210, f=w208) -> (s? t:f=w209:string)
              }
              frame 66 {
                # "lost qstation connection"
                n83 = call <vilib>:"Clear Errors.vi"("error in (no error)"=w215) -> ("error out"=w217:errorcluster)  [unwired: 5 in, 1 out]
              }
            }
          }
        }
        "LAST ERROR" <- w160
        n84 = call <vilib>:"Add State(s) to Queue__JKI_lib_State_Machine.vi"("State(s) in Front (\"\")"=w168) -> ("States Out"=w170:string)  [unwired: 14 in]
      }
      frame "Exit" {
        # "Do not put any code in this frame.\n(No errors that occur here will be handled.)"
        n85 = call <vilib>:"Add State(s) to Queue__JKI_lib_State_Machine.vi"("State(s) in (\"\")"=w222) -> ("States Out"=w221:string)  [unwired: 14 in]
      }
      frame "---------- Data ----------" {
        # "Do not put any code in this frame.\n(It is a separator no-op. You can make a copy of this frame to create a new Data frame)"
        n86 = call <vilib>:"Add State(s) to Queue__JKI_lib_State_Machine.vi"("State(s) in (\"\")"=w226) -> ("States Out"=w225:string)  [unwired: 14 in]
      }
      frame "Data: Initialize" {
        w228 = enum16{"online", "demo", "compile"}."online"  # mode
        w230 = 0.0  # winch parameter
        w231 = ""  # channel name
        w232 = T11."open/close=1/0"  # digital logic
        w233 = 0.0  # timeout
        w234 = 0.0  # time1
        w235 = T14 {"Current VI Reference"=refnum, "Close Panel on Exit?"=FALSE}  # Core
        # "do not delete - used by framework"
        # "Expand Bundle to add new data elements to shift register data."
        # "Data names and types of shift register data are defined by this bundle."
        # "Initialize the shift-register data, here.\n(data names are defined by what you wire into the bundle function)"
        n87 = control-ref of="proceed button"() -> (w229:refnum<vi>)
        n88 = control-ref of="Mode Tab"() -> (w227:refnum<vi>)
        n89 = Bundle("Core"=w235, "time1"=w234, "timeout"=w233, "digital logic"=w232, "channel name"=w231, "winch parameter"=w230, "proceed button"=w229, "Mode Tab"=w227, "mode"=w228) -> (w237:T12)  [unwired: 1 in]
        n90 = call <vilib>:"Add State(s) to Queue__JKI_lib_State_Machine.vi"("State(s) in (\"\")"=w239) -> ("States Out"=w238:string)  [unwired: 14 in]
      }
      frame "Data: Cleanup" {
        # "Cleanup any data and references, here.\n(this is called automatically, by the Macro: Exit)"
        n91 = Unbundle By Name(w240) -> ("Core.Current VI Reference"=w243:refnum<vi>)
        n92 = Close Reference(reference=w243, error in (no error)=w242) -> (error out=w241:errorcluster)
        n93 = call <vilib>:"Add State(s) to Queue__JKI_lib_State_Machine.vi"("State(s) in (\"\")"=w245) -> ("States Out"=w244:string)  [unwired: 14 in]
      }
      frame "---------- UI ----------" {
        # "Do not put any code in this frame.\n(It is a separator no-op. You can make a copy of this frame to create a new UI frame)"
        n94 = call <vilib>:"Add State(s) to Queue__JKI_lib_State_Machine.vi"("State(s) in (\"\")"=w249) -> ("States Out"=w248:string)  [unwired: 14 in]
      }
      frame "UI: Initialize" {
        # "Initialize the User Interface, here.\n(this is called automatically, by the Macro: Init)"
        n95 = call <vilib>:"Add State(s) to Queue__JKI_lib_State_Machine.vi"("State(s) in Front (\"\")"="UI: All Tabs >> Disable\nPrivate: Gauge Panel\nPrivate: Control Panel", "State(s) in (\"\")"=w254) -> ("States Out"=w253:string)  [unwired: 13 in]
      }
      frame "UI: Cursor Set" {
        # "Argument"
        # "Set and Unset Cursor Busy.\n(Usage: \"UI: Cursor Set >> Busy|Idle\")"
        n96 = case shown="\"idle\", Default" w255 {
          tunnel: w257 -> [w262 w264]
          tunnel: [w261 w263] -> w256
          frame "idle", Default {
            n97 = call <vilib>:"Unset Busy.vi"("error in (no error)"=w262) -> ("error out"=w261:errorcluster)  [unwired: 10 in]
          }
          frame "busy" {
            n98 = call <vilib>:"Set Busy.vi"("error in (no error)"=w264) -> ("error out"=w263:errorcluster)  [unwired: 9 in, 1 out]
          }
        }
        n99 = call <vilib>:"Add State(s) to Queue__JKI_lib_State_Machine.vi"("State(s) in (\"\")"=w260) -> ("States Out"=w259:string)  [unwired: 14 in]
      }
      frame "UI: Front Panel State" {
        # "Argument"
        # "Set Front Panel Open or Closed\n(Usage: \"UI: Front Panel State >> Open|Close\")"
        n100 = Unbundle By Name(w267) -> ("Core.Current VI Reference"=w266:refnum<vi>)
        n101 = case shown="\"open\", \"standard\", Default" w265 {
          tunnel: w269 -> [w277 w292 w303 w316 w329]
          tunnel: [w279 w293 w305 w318 w331] -> w268
          tunnel: w266 -> [w278 w290 w304 w317 w330]
          frame "open", "standard", Default {
            w272 = T6."Standard" ("State")
            n102 = property class="VI"(reference=w278, error in=w277) -> (reference out=w275:refnum<vi>, error out=w276:errorcluster, "FP.State"=w274:T6)
            n103 = Not Equal?(x=w274, y=w272) -> (x != y?=w273:bool)
            n104 = case shown="True" w273 {
              tunnel: [w283 w285] -> w279
              tunnel: w276 -> [w282 w285]
              tunnel: w275 -> [w281 _]
              tunnel: w272 -> [w280 _]
              frame True {
                n105 = invoke class="VI" method="FP.Open"(reference=w281, error in=w282, "Activate"=TRUE, "State"=w280) -> (error out=w283:errorcluster)  [unwired: 1 in, 4 out]
              }
              frame False {
              }
            }
          }
          frame "close", "closed" {
            n106 = property class="VI"(reference=w290, error in=w292) -> (reference out=w289:refnum<vi>, error out=w291:errorcluster, "FP.State"=w287:T6)
            n107 = Not Equal?(x=w287, y=T6."Closed" ("Front Panel Window:State")) -> (x != y?=w286:bool)
            n108 = case shown="True" w286 {
              tunnel: [w294 w297] -> w293
              tunnel: w291 -> [w294 w296]
              tunnel: w289 -> [_ w295]
              frame False {
              }
              frame True {
                n109 = invoke class="VI" method="FP.Close"(reference=w295, error in=w296) -> (error out=w297:errorcluster)  [unwired: 1 in, 2 out]
              }
            }
          }
          frame "hidden", "hide" {
            w298 = T6."Hidden" ("State")
            n110 = property class="VI"(reference=w304, error in=w303) -> (reference out=w301:refnum<vi>, error out=w302:errorcluster, "FP.State"=w300:T6)
            n111 = Not Equal?(x=w300, y=w298) -> (x != y?=w299:bool)
            n112 = case shown="True" w299 {
              tunnel: [w309 w310] -> w305
              tunnel: w302 -> [w308 w310]
              tunnel: w301 -> [w307 _]
              tunnel: w298 -> [w306 _]
              frame True {
                n113 = invoke class="VI" method="FP.Open"(reference=w307, error in=w308, "State"=w306) -> (error out=w309:errorcluster)  [unwired: 2 in, 4 out]
              }
              frame False {
              }
            }
          }
          frame "minimize", "minimized" {
            w311 = T6."Minimized" ("State")
            n114 = property class="VI"(reference=w317, error in=w316) -> (reference out=w314:refnum<vi>, error out=w315:errorcluster, "FP.State"=w313:T6)
            n115 = Not Equal?(x=w313, y=w311) -> (x != y?=w312:bool)
            n116 = case shown="True" w312 {
              tunnel: [w322 w323] -> w318
              tunnel: w315 -> [w321 w323]
              tunnel: w314 -> [w320 _]
              tunnel: w311 -> [w319 _]
              frame True {
                n117 = invoke class="VI" method="FP.Open"(reference=w320, error in=w321, "State"=w319) -> (error out=w322:errorcluster)  [unwired: 2 in, 4 out]
              }
              frame False {
              }
            }
          }
          frame "maximize", "maximized" {
            w324 = T6."Maximized" ("State")
            n118 = property class="VI"(reference=w330, error in=w329) -> (reference out=w327:refnum<vi>, error out=w328:errorcluster, "FP.State"=w326:T6)
            n119 = Not Equal?(x=w326, y=w324) -> (x != y?=w325:bool)
            n120 = case shown="True" w325 {
              tunnel: [w335 w336] -> w331
              tunnel: w328 -> [w334 w336]
              tunnel: w327 -> [w333 _]
              tunnel: w324 -> [w332 _]
              frame True {
                n121 = invoke class="VI" method="FP.Open"(reference=w333, error in=w334, "State"=w332) -> (error out=w335:errorcluster)  [unwired: 2 in, 4 out]
              }
              frame False {
              }
            }
          }
        }
        n122 = call <vilib>:"Add State(s) to Queue__JKI_lib_State_Machine.vi"("State(s) in (\"\")"=w271) -> ("States Out"=w270:string)  [unwired: 14 in]
      }
      frame "UI: Proceed Button" {
        # "Enable/Disable the \"Proceed\" UI button\n(the button value affects \"Wait...\" states)"
        n123 = Unbundle By Name(w340) -> ("proceed button"=w339:refnum<vi>, "mode"=w338:enum16{"online", "demo", "compile"})
        n124 = case shown="\"online\", \"demo\", Default" w338 {
          tunnel: [TRUE ("Blinking") FALSE ("Blinking")] -> w337
          frame "compile" {
          }
          frame "online", "demo", Default {
          }
        }
        n125 = case shown="\"disable\"" w343 {
          tunnel: w339 -> [w351 w357]
          tunnel: w342 -> [w350 w359]
          tunnel: [w349 w358] -> w341
          tunnel: w337 -> [w348 w354]
          frame "disable" {
            n126 = property class="Bool (strict)"(reference=w351, error in=w350, "Blinking"=FALSE ("Value"), "DisabledEnum"=T8."Disabled and Grayed Out" ("Disabled"), "Value"=w348) -> (error out=w349:errorcluster)  [unwired: 1 out]
          }
          frame "enable", Default {
            n127 = property class="Bool (strict)"(reference=w357, error in=w359, "Blinking"=TRUE ("Value"), "DisabledEnum"=T8."Enabled" ("Disabled"), "Value"=w354) -> (error out=w358:errorcluster)  [unwired: 1 out]
          }
        }
        n128 = call <vilib>:"Add State(s) to Queue__JKI_lib_State_Machine.vi"("State(s) in (\"\")"=w345) -> ("States Out"=w344:string)  [unwired: 14 in]
      }
      frame "UI: Pause Button" {
        # "Wait until Proceed Button is hit, then start auto sequence\n(This is called from \"Idle\" state)"
        n129 = case shown="\"disable\"" w362 {
          tunnel: [T8."Disabled and Grayed Out" ("Disabled") T8."Enabled" ("Disabled")] -> w361
          frame "disable" {
          }
          frame "enable", Default {
          }
        }
        n130 = control-ref of="pause button"() -> (w363:refnum<vi>)
        n131 = property class="Bool (strict)"(reference=w363, "DisabledEnum"=w361, "Value"=FALSE) -> ()  [unwired: 1 in, 2 out]
        n132 = Wait (ms)(milliseconds to wait=u32 50) -> ()  [unwired: 1 out]
        n133 = call <vilib>:"Add State(s) to Queue__JKI_lib_State_Machine.vi"("State(s) in (\"\")"=w368) -> ("States Out"=w367:string)  [unwired: 14 in]
      }
      frame "UI: Return Button" {
        # "Wait until Proceed Button is hit, then start auto sequence\n(This is called from \"Idle\" state)"
        n134 = case shown="\"enable\", Default" w372 {
          tunnel: [T8."Disabled and Grayed Out" ("Disabled") T8."Enabled" ("Disabled")] -> w371
          frame "disable" {
          }
          frame "enable", Default {
          }
        }
        n135 = control-ref of="return button"() -> (w373:refnum<vi>)
        n136 = property class="Bool"(reference=w373, "DisabledEnum"=w371) -> ()  [unwired: 1 in, 2 out]
        n137 = Wait (ms)(milliseconds to wait=u32 50) -> ()  [unwired: 1 out]
        n138 = call <vilib>:"Add State(s) to Queue__JKI_lib_State_Machine.vi"("State(s) in (\"\")"=w378) -> ("States Out"=w377:string)  [unwired: 14 in]
      }
      frame "UI: One Tab Enable" {
        # "Enables the tab passed as an argument\n(zero-indexed, from left to right)"
        n139 = Unbundle By Name(w385) -> ("Mode Tab"=w381:refnum<vi>)
        n140 = Decimal String To Number(string=w387) -> (number=w386:i32)  [unwired: 2 in, 1 out]
        n141 = property class="TabCtl (strict)"(reference=w381, error in=w384, "DisabledEnum"=T8."Enabled" ("Disabled")) -> (error out=w383:errorcluster, "Pages"=w388:refnum<vi>[])  [unwired: 1 out]
        n142 = for {
          tunnel: w388 -> [w395] mode=indexing
          tunnel: w386 -> [w393]
          i -> [w394]
          # "one tab"
          n143 = Equal?(x=w393, y=w394) -> (x = y?=w392:bool)
          n144 = case shown="True" w392 {
            tunnel: w395 -> [_ w397]
            frame False {
            }
            frame True {
              n145 = property class="Page"(reference=w397, "PageEnb"=T9."Page Enabled" ("Page Enabled State")) -> ()  [unwired: 1 in, 2 out]
            }
          }
        }
        n146 = Wait (ms)(milliseconds to wait=u32 50) -> ()  [unwired: 1 out]
        n147 = call <vilib>:"Add State(s) to Queue__JKI_lib_State_Machine.vi"("State(s) in (\"\")"=w391) -> ("States Out"=w390:string)  [unwired: 14 in]
      }
      frame "UI: Change Tabs" {
        # "Sets the active tab based on the argument passed\n(zero-indexed, from left to right)"
        n148 = Decimal String To Number(string=w401) -> (number=w399:i32)  [unwired: 2 in, 1 out]
        n149 = Unbundle By Name(w400) -> ("Mode Tab"=w398:refnum<vi>)
        n150 = property class="TabCtl (strict)"(reference=w398, "Value"=w399) -> ()  [unwired: 1 in, 2 out]
        n151 = call <vilib>:"Add State(s) to Queue__JKI_lib_State_Machine.vi"("State(s) in (\"\")"=w404) -> ("States Out"=w403:string)  [unwired: 14 in]
      }
      frame "UI: All Tabs" {
        # "Wait until Proceed Button is hit, then start auto sequence\n(This is called from \"Idle\" state)"
        n152 = case shown="\"enable\", Default" w409 {
          tunnel: [T9."Page Disabled & Grayed" ("Page Enabled State") T9."Page Enabled" ("Page Enabled State")] -> w408
          tunnel: [T8."Disabled and Grayed Out" ("Disabled") T8."Enabled" ("Disabled")] -> w406
          frame "disable" {
          }
          frame "enable", Default {
          }
        }
        n153 = control-ref of="Mode Tab"() -> (w405:refnum<vi>)
        n154 = property class="TabCtl (strict)"(reference=w405, "DisabledEnum"=w406) -> ("Pages"=w407:refnum<vi>[])  [unwired: 1 in, 2 out]
        n155 = for {
          tunnel: w408 -> [w416]
          tunnel: w407 -> [w415] mode=indexing
          # "all tabs"
          n156 = property class="Page"(reference=w415, "PageEnb"=w416) -> ()  [unwired: 1 in, 2 out]
        }
        n157 = Wait (ms)(milliseconds to wait=u32 50) -> ()  [unwired: 1 out]
        n158 = call <vilib>:"Add State(s) to Queue__JKI_lib_State_Machine.vi"("State(s) in (\"\")"=w414) -> ("States Out"=w413:string)  [unwired: 14 in]
      }
      frame "---------- Macro ----------" {
        # "Do not put any code in this frame.\n(It is a separator no-op. You can make a copy of this frame to create a new Macro frame)"
        n159 = call <vilib>:"Add State(s) to Queue__JKI_lib_State_Machine.vi"("State(s) in (\"\")"=w424) -> ("States Out"=w423:string)  [unwired: 14 in]
      }
      frame "ENTRY: Standby" {
        # "Set up UI and prepare to enter \"Standby\" tab"
        n160 = Wait (ms)(milliseconds to wait=u32 50) -> ()  [unwired: 1 out]
        n161 = call <vilib>:"Add State(s) to Queue__JKI_lib_State_Machine.vi"("State(s) in Front (\"\")"="STATUS >> Standby\nACT_EMATCH >> Off\nACT_SIREN >> Off\nPrivate: Winch action >> Off\nUI: Return Button >> Disable\nUI: Pause Button >> Disable\nUI: Proceed Button >> Disable\nUI: All Tabs >> Enable\nUI: Change Tabs >> 0\nPrivate: Sub Panel Control Panel >> Disable\nIdle", "State(s) in (\"\")"=w430) -> ("States Out"=w429:string)  [unwired: 13 in]
      }
      frame "Macro: Default DAQ Output" {
        # "Initialization Macro\n(This is called once, when the VI starts)"
        n162 = call <vilib>:"Add State(s) to Queue__JKI_lib_State_Machine.vi"("State(s) in Front (\"\")"="ACT_FILL_FU >> Close\nACT_FILL_OX >> Close\nACT_MAIN_FU >> Close\nACT_MAIN_OX >> Close\nACT_MBV >> Close\nACT_PRESS_FU >> Close\nACT_PRESS_OX >> Close\nACT_PURGE_FU >> Close\nACT_PURGE_OX  >> Close\nACTI_VENT_FU >> Open\nACTI_VENT_OX >> Open\nACT_EMATCH >> Off\nACT_SIREN >> Off\nACT_WINCH_ON >> Off\nLOG_TRIG_ON >> Off\nDAQ_ARM >> On", "State(s) in (\"\")"=w435) -> ("States Out"=w434:string)  [unwired: 13 in]
      }
      frame "ENTRY: Auto Sequence" {
        # "Set up UI and prepare to start Auto Sequence"
        n163 = Wait (ms)(milliseconds to wait=u32 50) -> ()  [unwired: 1 out]
        n164 = call <vilib>:"Add State(s) to Queue__JKI_lib_State_Machine.vi"("State(s) in Front (\"\")"="Private: Check Gauge Panel Errors\nACT_EMATCH >> Off\nACT_SIREN >> Off\nPrivate: Winch action >> Off\nUI: All Tabs >> Disable\nUI: One Tab Enable >> 2\nUI: Change Tabs >> 2\n//UI: Proceed Button >> Enable\n//Private: Wait for Proceed Button\nMacro: INIT SubVIs >> Compile\nSTATUS >> Starting offline compilation... (no commands will be sent)\nMacro: Add States from Text File >> Auto //run through all states in demo mode to expose any errors \nMacro: INIT SubVIs >> Online\nUI: Proceed Button >> Enable\nUI: Return Button >> Enable\nUI: Pause Button >> Enable\nSTATUS >> Compilation passed! Press \"Proceed\" to start Auto Sequence\nPrivate: Wait for Proceed Button //get user consent before proceeding\nMacro: Add States from Text File >> Auto //run for real\nENTRY: Standby", "State(s) in (\"\")"=w437) -> ("States Out"=w441:string)  [unwired: 13 in]
      }
      frame "ENTRY: Commands File" {
        # "Set up UI and prepare to start Auto Sequence"
        n165 = Wait (ms)(milliseconds to wait=u32 50) -> ()  [unwired: 1 out]
        n166 = call <vilib>:"Add State(s) to Queue__JKI_lib_State_Machine.vi"("State(s) in Front (\"\")"="Private: Check Gauge Panel Errors\nACT_EMATCH >> Off\nACT_SIREN >> Off\nPrivate: Winch action >> Off\nUI: All Tabs >> Disable\nUI: One Tab Enable >> 2\nUI: Change Tabs >> 2\n//UI: Proceed Button >> Enable\n//Private: Wait for Proceed Button\nMacro: INIT SubVIs >> Compile\nSTATUS >> Starting offline compilation... (no commands will be sent)\nMacro: Add States from Text File >> Auto //run through all states in demo mode to expose any errors \nMacro: INIT SubVIs >> Online\nUI: Proceed Button >> Enable\nUI: Return Button >> Enable\nUI: Pause Button >> Enable\nSTATUS >> Compilation passed! Press \"Proceed\" to start Auto Sequence\nPrivate: Wait for Proceed Button //get user consent before proceeding\nMacro: Add States from Text File >> Auto //run for real\nENTRY: Standby", "State(s) in (\"\")"=w443) -> ("States Out"=w447:string)  [unwired: 13 in]
      }
      frame "Macro: Add States from Text File" {
        # "Run a list of commands from a text file"
        n167 = case shown="Default" w448 {
          tunnel: ["CLEANUP_PROCEDURE_COMMANDS.txt" ("name or relative path") "lol.lol" ("name or relative path") "AUTO_SEQUENCE_COMMANDS.txt" ("name or relative path")] -> w451
          frame "cleanup" {
          }
          frame Default {
            # "dummy"
          }
          frame "auto" {
          }
        }
        n168 = call <vilib>:"Application Directory.vi"() -> ("Application Directory"=w452:path)
        n169 = Build Path(base path=w452, name or relative path=w451) -> (appended path=w453:path)
        n170 = call <vilib>:"Check if File or Folder Exists.vi"("path"=w453) -> ("file or folder exists?"=w454:bool)  [unwired: 8 in, 2 out]
        n171 = case shown="False" w454 {
          tunnel: w453 -> [_ w470]
          tunnel: [w464 w469] -> w449
          tunnel: [w463 FALSE ("cancelled")] -> w450
          frame False {
            n172 = Read from Text File(prompt (Open existing file)="Please select the COMMANDS text file for this test", count=-1) -> (text=w464:string, cancelled=w463:bool)  [unwired: 2 in, 2 out]
          }
          frame True {
            n173 = Read from Text File(file (use dialog)=w470, count=-1) -> (text=w469:string)  [unwired: 2 in, 3 out]
          }
        }
        n174 = case shown="True" w450 {
          tunnel: w456 -> [w471 w473]
          tunnel: [w471 w474] -> w455
          frame False {
          }
          frame True {
            w476 = 42 items=["No error", "Argument error", "Memory is full", "Out of zone", "End of file", "File already open", "Generic file I/O error", "File not found", "File permission error", "Disk is full", "Duplicate path", "Too many files open", "System feature not enabled", "Resource file not found", "Cannot add resource", "Resource not found", "Image not found", "Image memory error", "Pen does not exist", "Config type invalid", "Config token not found", "Config parse error", "Config memory error", "Bad external code format", "Bad external code offset", "External code not present", "Null window", "Destroy window error", "Null menu", "Print aborted", "Bad print record", "Print driver error", "Windows error during printing", "Memory error during printing", "Print dialog error", "Generic print error", "Invalid device refnum", "Device not found", "Device parameter error", "Device unit error", "Cannot open device", "Device call aborted", "Generic error", "Cancelled by user", "Object ID too low", "Object ID too high", "Object not in heap", "Unknown heap", "Unknown object (invalid DefProc)", "Unknown object (DefProc not in table)", "Message out of range", "Invalid (null) method", "Unknown message", "Manager call not supported", "Bad address", "Network operation in progress", "Network operation timed out", "Connection is busy", "Network attribute not supported", "Network error", "Address in use", "System out of memory", "Connection aborted", "Connection refused", "Not connected", "Already connected", "Connection closed", "Initialization error (interapplication manager)", "Bad occurrence", "Wait on unbound occurrence handler", "Occurrence queue overflow", "Datalog type conflict", "Unused", "Unrecognized type (interapplication manager)", "Memory corrupt", "Failed to make temporary DLL", "Old CIN version", "Drag socket not found", "Failed to load drop-object", "Failed to register OLE object", "Failed to release OLE object", "Format specifier type mismatch", "Unknown format specifier", "Too few format specifiers", "Too many format specifiers", "Scan failed", "Newer CIN version", "Error converting to variant", "Runtime menu error", "Password tampered", "Variant attribute not found", "Incompatible variant data type", "Event data is not available", "Event Store is not present", "Occurrence is not found", "Event Queue is not created", "Event info is not available", "Refnum passed is NULL", "Error retrieving Class GUID", "Error retrieving CoClass GUID", "Error retrieving TypeLib GUID.", "Bad built application magic bytes.", "Specific driver is different from the specific driver associated with the Logical Name.", "There is no session opened to the class driver.", "Max Error", "MAX - Error with config objects", "MAX - Error loading configuration", "MAX - Group not supported"]
            n175 = call <vilib>:"Error Cluster From Error Code.vi"("show call chain? (False)"=TRUE, "error in (no error)"=w473, "error message (\"\")"="Software Exception: could not load Auto Sequence Commands text file" ("message"), "error code (0)"=w476) -> ("error out"=w474:errorcluster)  [unwired: 5 in]
          }
        }
        n176 = call <vilib>:"Add State(s) to Queue__JKI_lib_State_Machine.vi"("State(s) in Front (\"\")"=w449, "State(s) in (\"\")"=w459) -> ("States Out"=w458:string)  [unwired: 13 in]
      }
      frame "Private: Check Gauge Panel Errors" {
        # "Run a list of commands from a text file"
        n177 = global read "global_variable_GAUGE_PANEL_ERROR.vi" "GAUGE PANEL ERROR"() -> (w480:bool)
        n178 = case shown="True" w480 {
          tunnel: ["Private: no-op" ("T button name (\"OK\")") w485] -> w479
          tunnel: w477 -> [_ w484]
          frame False {
          }
          frame True {
            n179 = Two Button Dialog(message="ERROR: Check  GAUGE PANEL for sensors that are out-of-range.", 1:"Proceed Anyway (NOT RECOMMENDED)" ("F button name (\"Cancel\")"), 2:"Return to Standby" ("T button name (\"OK\")")) -> (T button?=w487:bool)
            n180 = Select(t="ENTRY: Standby" ("T button name (\"OK\")"), s=w487, f=w484) -> (s? t:f=w485:string)
          }
        }
        n181 = call <vilib>:"Add State(s) to Queue__JKI_lib_State_Machine.vi"("State(s) in Front (\"\")"=w479) -> ("States Out"=w482:string)  [unwired: 14 in]
      }
      frame "ENTRY: Control Panel" {
        # "Set up UI and prepare to start Auto Sequence"
        n182 = Wait (ms)(milliseconds to wait=u32 50) -> ()  [unwired: 1 out]
        n183 = call <vilib>:"Add State(s) to Queue__JKI_lib_State_Machine.vi"("State(s) in Front (\"\")"="STATUS >> You can now actuate\nACT_EMATCH >> Off\nACT_SIREN >> Off\nPrivate: Winch action >> Off\nUI: Proceed Button >> Disable\nUI: Return Button >> Enable\nUI: Pause Button >> Disable\nUI: All Tabs >> Disable\nUI: One Tab Enable >> 1\nUI: Change Tabs >> 1\nPrivate: Sub Panel Control Panel >> Enable\nPrivate: Wait for Proceed Button // this keeps us from returning to Idle state", "State(s) in (\"\")"=w492) -> ("States Out"=w496:string)  [unwired: 13 in]
      }
      frame "Private: Control Panel" {
        w501 = 128  # call and forget
        # "Asyncronous call to virtual_control_box.vi subvi.\nState will move on without waiting for results."
        # "Set up UI and prepare to start Auto Sequence"
        n184 = vi-ref "control_panel.vi"() -> (w500:refnum<vi>)
        n185 = invoke on="Sub Panel - Control Panel" class="SubPnl" method="Insert VI"("VI Ref"=w500) -> ()  [unwired: 3 in, 4 out]
        n186 = property class="VI"(reference=w500, error in=w499) -> (error out=w507:errorcluster, "Name"=w506:string)  [unwired: 1 out]
        n187 = Open VI Reference(type specifier VI Refnum (for type only)=refnum<vi> refnum, vi path=w506, options=w501, error in (no error)=w507) -> (vi reference=w503:refnum<vi>, error out=w504:errorcluster)  [unwired: 2 in]
        n188 = call-by-ref "Start Asynchronous Call"(reference=w503, error in=w504) -> (reference out=w508:refnum<vi>, error out=w505:errorcluster)  [unwired: 12 in]
        n189 = Close Reference(reference=w508, error in (no error)=w505) -> (error out=w498:errorcluster)
        n190 = call <vilib>:"Add State(s) to Queue__JKI_lib_State_Machine.vi"("State(s) in Front (\"\")"=w497) -> ("States Out"=w510:string)  [unwired: 14 in]
      }
      frame "Private: Sub Panel Control Panel" {
        # "Set up UI and prepare to start Auto Sequence"
        n191 = case shown="\"disable\", Default" w512 {
          frame "disable", Default {
            n192 = property on="Sub Panel" class="SubPnl"("DisabledEnum"=T8."Disabled" ("Disabled")) -> ()  [unwired: 2 in, 2 out]
          }
          frame "enable" {
            n193 = property on="Sub Panel" class="SubPnl"("DisabledEnum"=T8."Enabled" ("Disabled")) -> ()  [unwired: 2 in, 2 out]
          }
        }
        n194 = call <vilib>:"Add State(s) to Queue__JKI_lib_State_Machine.vi"("State(s) in Front (\"\")"=w513) -> ("States Out"=w515:string)  [unwired: 14 in]
      }
      frame "ENTRY: Cleanup Procedure" {
        # "Set up UI and prepare to start Auto Sequence"
        n195 = Wait (ms)(milliseconds to wait=u32 50) -> ()  [unwired: 1 out]
        n196 = call <vilib>:"Add State(s) to Queue__JKI_lib_State_Machine.vi"("State(s) in Front (\"\")"="LOG_TRIG_ON >> Off\nACT_EMATCH >> Off\nACT_SIREN >> Off\nPrivate: Winch action >> Off\nUI: Proceed Button >> Enable\nUI: Return Button >> Enable\nUI: Pause Button >> Enable\nUI: All Tabs >> Disable\nUI: One Tab Enable >> 3\nUI: Change Tabs >> 3\nPrivate: Wait for Proceed Button\nUI: Proceed Button >> Disable\nMacro: INIT SubVIs >> Demo\nMacro: Add States from Text File >> Cleanup //run through all states in demo mode to expose any errors \nMacro: INIT SubVIs\nMacro: Add States from Text File >> Cleanup  //run for real", "State(s) in (\"\")"=w519) -> ("States Out"=w523:string)  [unwired: 13 in]
      }
      frame "Private: Gauge Panel" {
        w528 = 128  # call and forget
        # "Asyncronous call to virtual_gauge_panel subvi.\nState will move on without waiting for results."
        # "Set up UI and prepare to start Auto Sequence"
        n197 = vi-ref "gauge_panel.vi"() -> (w524:refnum<vi>)
        n198 = property class="VI"(reference=w524, error in=w527) -> (error out=w534:errorcluster, "Name"=w533:string)  [unwired: 1 out]
        n199 = invoke on="Sub Panel - Gauge Panel" class="SubPnl" method="Insert VI"("VI Ref"=w524) -> ()  [unwired: 3 in, 4 out]
        n200 = Open VI Reference(type specifier VI Refnum (for type only)=refnum<vi> refnum, vi path=w533, options=w528, error in (no error)=w534) -> (vi reference=w530:refnum<vi>, error out=w531:errorcluster)  [unwired: 2 in]
        n201 = call-by-ref "Start Asynchronous Call"(reference=w530, error in=w531) -> (reference out=w535:refnum<vi>, error out=w532:errorcluster)  [unwired: 12 in]
        n202 = Close Reference(reference=w535, error in (no error)=w532) -> (error out=w526:errorcluster)
        n203 = call <vilib>:"Add State(s) to Queue__JKI_lib_State_Machine.vi"("State(s) in Front (\"\")"=w525) -> ("States Out"=w537:string)  [unwired: 14 in]
      }
      frame "Macro: INIT SubVIs" {
        w556 = "" ("channel")
        w554 = TRUE ("INIT?")
        # "run this because in \"compile\" mode\nproceed button will be forced TRUE\nso there is never waiting"
        # "initialize these 3 subVIs"
        # "dummies for required inputs"
        # "Initialization Macro\n(This is called once, when the VI starts)"
        n204 = case shown="True" "demo mode" {
          tunnel: w553 -> [w614 w618]
          tunnel: [w613 w619] -> w547
          frame False {
            n205 = case shown="\"online\", Default" w614 {
              tunnel: [enum16{"online", "demo", "compile"}."online" ("INIT mode") enum16{"online", "demo", "compile"}."demo" ("INIT mode") enum16{"online", "demo", "compile"}."compile" ("INIT mode")] -> w613
              frame "online", Default {
              }
              frame "demo" {
              }
              frame "compile" {
              }
            }
          }
          frame True {
            n206 = case shown="\"demo\", \"online\", Default" w618 {
              tunnel: [enum16{"online", "demo", "compile"}."demo" ("INIT mode") enum16{"online", "demo", "compile"}."compile" ("INIT mode")] -> w619
              frame "demo", "online", Default {
              }
              frame "compile" {
              }
            }
          }
        }
        n207 = case shown="\"compile\"" w547 {
          selector: w547 -> [w562 w565 w589]
          tunnel: w550 -> [w561 w573 w595]
          tunnel: [_ w569 w591] -> w549
          tunnel: [w561 w568 w593] -> w540
          tunnel: [w562 w567 w590] -> w543
          tunnel: "DAQ IP Address" -> [_ w566 w588]
          tunnel: "demo mode" -> [_ _ w587]
          tunnel: ["UI: Proceed Button >> Disable" ("State(s) in Front (\"\")") w563 w586] -> w539
          frame "demo" {
          }
          frame "online", Default {
            w572 = 0  # Buffer Index
            w574 = e.gate_Protocol_Type."HighspeedPort Online"  # Protocol
            # "Connect to QSTATION"
            n208 = call <instrlib>:"e.gate Initialize.vi"("Buffer Index"=w572, "error in (no error)"=w573, "Protocol"=w574, "IP Address"=w566) -> ("error out"=w570:errorcluster, "e.gate Configuration"=w571:T16)  [unwired: 6 in]
            n209 = case shown="Error" w570 {
              selector: w570 -> [w577 w580]
              tunnel: [w578 w581] -> w569
              tunnel: w571 -> [w578 w581]
              tunnel: [w577 w579] -> w568
              tunnel: [w576 w582] -> w567
              tunnel: w565 -> [w576 w582]
              tunnel: "NOTICE: No connection to QSTATION.\nRetrying" ("channel") -> [_ w584]
              tunnel: ["UI: Proceed Button >> Disable" ("State(s) in Front (\"\")") "Macro: INIT SubVIs >> Online" ("channel")] -> w563
              frame No Error {
              }
              frame Error {
                # "force retry"
                n210 = One Button Dialog(message=w584) -> ()  [unwired: 1 in, 1 out]
                n211 = call <vilib>:"Clear Errors.vi"("error in (no error)"=w580) -> ("error out"=w579:errorcluster)  [unwired: 5 in, 1 out]
              }
            }
          }
          frame "compile" {
            n212 = case shown="True" w587 {
              tunnel: w595 -> [w599 _]
              tunnel: [w598 w603] -> w594
              tunnel: [w597 _] -> w592
              tunnel: w588 -> [w596 _]
              frame False {
                w600 = 0  # Buffer Index
                w601 = e.gate_Protocol_Type."HighspeedPort Online"  # Protocol
                # "Connect to QSTATION"
                n213 = call <instrlib>:"e.gate Initialize.vi"("Buffer Index"=w600, "error in (no error)"=w599, "Protocol"=w601, "IP Address"=w596) -> ("error out"=w598:errorcluster, "e.gate Configuration"=w597:T16)  [unwired: 6 in]
              }
              frame True {
                n214 = call <vilib>:"Error Cluster From Error Code.vi"("error code (0)"=1) -> ("error out"=w603:errorcluster)  [unwired: 8 in]
              }
            }
            n215 = case shown="Error" w594 {
              selector: w594 -> [w607 w609]
              tunnel: [w607 w608] -> w593
              tunnel: w592 -> [w606 _]
              tunnel: [w606 _] -> w591
              tunnel: w589 -> [w605 w612]
              tunnel: [w605 w612] -> w590
              tunnel: "NOTICE: No connection to QSTATION." ("channel") -> [_ w611]
              tunnel: ["UI: Proceed Button >> Disable" ("State(s) in Front (\"\")") "Macro: INIT SubVIs >> Online" ("channel")] -> w586
              frame No Error {
              }
              frame Error {
                n216 = call <vilib>:"Clear Errors.vi"("error in (no error)"=w609) -> ("error out"=w608:errorcluster)  [unwired: 5 in, 1 out]
                n217 = One Button Dialog(message=w611) -> ()  [unwired: 1 in, 1 out]
              }
            }
          }
        }
        n218 = call "daq_output.vi"("INIT e.gate Configuration"=w549, "INIT mode"=w543, "INIT? (F)"=w554, "value"=0.0, "channel"=w556) -> ("error out"=w558:errorcluster)  [unwired: 6 in]
        n219 = call "daq_input.vi"("INIT e.gate Configuration"=w549, "INIT mode"=w543, "INIT? (F)"=w554, "error in (no error)"=w558, "channel"=w556) -> ("error out"=w555:errorcluster)  [unwired: 5 in, 1 out]
        n220 = Select(t=enum16{"online", "demo", "compile"}."demo" ("INIT mode"), s="ignore limit switch feedback", f=w543) -> (s? t:f=w544:enum16{"online", "demo", "compile"})
        n221 = call "fbk_timeout_error.vi"("INIT mode"=w544, "INIT? (F)"=w554, "error in (no error)"=w555) -> ("error out"=w541:errorcluster)  [unwired: 8 in]
        n222 = call <vilib>:"Clear Errors.vi"("error in (no error)"=w541) -> ()  [unwired: 5 in, 2 out]
        n223 = call <vilib>:"Add State(s) to Queue__JKI_lib_State_Machine.vi"("State(s) in Front (\"\")"=w539, "State(s) in (\"\")"=w538) -> ("States Out"=w559:string)  [unwired: 13 in]
        n224 = Bundle By Name(cluster=w552, "mode"=w543) -> (w551:T12)
      }
      frame "---------- Special Commands ----------" {
        # "Template Separator\n(You can make a copy of, or modify, this frame)"
        n225 = call <vilib>:"Add State(s) to Queue__JKI_lib_State_Machine.vi"("State(s) in (\"\")"=w625) -> ("States Out"=w624:string)  [unwired: 14 in]
      }
      frame "Calibration" {
        (unwired) "Winch >> Pull,100 //pull to 100LBF then turn off\nWait >> 0.5 //remain in off state for 0.5sec to settle\nWinch >> Pull,200\nWait >> 0.5\nWinch >> Pull,300\nWait >> 0.5\nWinch >> Pull,400\nWait >> 0.5\nWinch >> Release,-10 //release winch to -10LBF then turn off"
        # "Pull incrementally up to a certain force then release the winch"
        n226 = call <vilib>:"Add State(s) to Queue__JKI_lib_State_Machine.vi"("State(s) in Front (\"\")"="Winch >> Pull,250\nWait >> 1\nWinch >> Release,200\nWait >> 1\nWinch >> Release,150\nWait >> 1\nWinch >> Release,100\nWait >> 1\nWinch >> Release,0", "State(s) in (\"\")"=w627) -> ("States Out"=w630:string)  [unwired: 13 in]
      }
      frame "Winch" {
        # "the value that, if reached while releasing the winch,\nmeans the winch is actually pulling and needs to\nchange directions"
        # "Initial setup before actually actuating the winch\n(must be called before calling \"Private: Winch action\")"
        n227 = Match Pattern(string=w646, regular expression=",") -> (after substring=w656:string)  [unwired: 1 in, 3 out]
        n228 = Fract/Exp String To Number(string=w656) -> (number=w650:dbl)  [unwired: 3 in, 1 out]
        n229 = Less Or Equal?(x=w650, y=800.0) -> (x <= y?=w652:bool)
        n230 = Less Or Equal?(x=w650, y=-100.0) -> (x <= y?=w651:bool)
        n231 = call <vilib>:"Build State String with Arguments__JKI_lib_State_Machine.vi"("Arguments (\"\")"=w646, "State"="Private: Winch action") -> ("State with Arguments"=w638:string)  [unwired: 4 in]
        n232 = Or(x=w652, y=w651) -> (x .or. y?=w653:bool)
        n233 = call "daq_input.vi"("error in (no error)"=w644, "channel"="LOAD_CALIBRATION") -> ("error out"=w643:errorcluster, "value"=w645:dbl)  [unwired: 8 in]
        n234 = case shown="False" w653 {
          tunnel: w643 -> [w660 w666]
          tunnel: [w659 w666] -> w642
          tunnel: w650 -> [w658 _]
          frame False {
            w664 = 42 items=["No error", "Argument error", "Memory is full", "Out of zone", "End of file", "File already open", "Generic file I/O error", "File not found", "File permission error", "Disk is full", "Duplicate path", "Too many files open", "System feature not enabled", "Resource file not found", "Cannot add resource", "Resource not found", "Image not found", "Image memory error", "Pen does not exist", "Config type invalid", "Config token not found", "Config parse error", "Config memory error", "Bad external code format", "Bad external code offset", "External code not present", "Null window", "Destroy window error", "Null menu", "Print aborted", "Bad print record", "Print driver error", "Windows error during printing", "Memory error during printing", "Print dialog error", "Generic print error", "Invalid device refnum", "Device not found", "Device parameter error", "Device unit error", "Cannot open device", "Device call aborted", "Generic error", "Cancelled by user", "Object ID too low", "Object ID too high", "Object not in heap", "Unknown heap", "Unknown object (invalid DefProc)", "Unknown object (DefProc not in table)", "Message out of range", "Invalid (null) method", "Unknown message", "Manager call not supported", "Bad address", "Network operation in progress", "Network operation timed out", "Connection is busy", "Network attribute not supported", "Network error", "Address in use", "System out of memory", "Connection aborted", "Connection refused", "Not connected", "Already connected", "Connection closed", "Initialization error (interapplication manager)", "Bad occurrence", "Wait on unbound occurrence handler", "Occurrence queue overflow", "Datalog type conflict", "Unused", "Unrecognized type (interapplication manager)", "Memory corrupt", "Failed to make temporary DLL", "Old CIN version", "Drag socket not found", "Failed to load drop-object", "Failed to register OLE object", "Failed to release OLE object", "Format specifier type mismatch", "Unknown format specifier", "Too few format specifiers", "Too many format specifiers", "Scan failed", "Newer CIN version", "Error converting to variant", "Runtime menu error", "Password tampered", "Variant attribute not found", "Incompatible variant data type", "Event data is not available", "Event Store is not present", "Occurrence is not found", "Event Queue is not created", "Event info is not available", "Refnum passed is NULL", "Error retrieving Class GUID", "Error retrieving CoClass GUID", "Error retrieving TypeLib GUID.", "Bad built application magic bytes.", "Specific driver is different from the specific driver associated with the Logical Name.", "There is no session opened to the class driver.", "Max Error", "MAX - Error with config objects", "MAX - Error loading configuration", "MAX - Group not supported"]
            n235 = Format Into String(format string="Software Exception: You should not actuate the winch with %f LBF" ("message"), error in=w660, w658) -> (resulting string=w663:string, error out=w662:errorcluster)  [unwired: 1 in]
            n236 = call <vilib>:"Error Cluster From Error Code.vi"("show call chain? (False)"=TRUE, "error in (no error)"=w662, "error message (\"\")"=w663, "error code (0)"=w664) -> ("error out"=w659:errorcluster)  [unwired: 5 in]
          }
          frame True {
          }
        }
        n237 = Add(x=80.0, y=w645) -> (x+y=w641:dbl)
        n238 = Concatenate Strings("UI: Proceed Button >> Enable\nUI: Return Button >> Disable\nUI: Pause Button >> Disable", "\n", w638, "\n", "UI: Return Button >> Enable\nUI: Pause Button >> Enable\nUI: Proceed Button >> Disable") -> (w635:string)
        n239 = Bundle By Name(cluster=w633, "winch parameter"=w641) -> (w640:T12)
        n240 = call <vilib>:"Add State(s) to Queue__JKI_lib_State_Machine.vi"("State(s) in Front (\"\")"=w635, "State(s) in (\"\")"=w634) -> ("States Out"=w657:string)  [unwired: 13 in]
      }
      frame "Private: Winch action" {
        # "Winch control\n(must be called by \"Winch\")"
        n241 = Unbundle By Name(w673) -> ("winch parameter"=w674:dbl, "proceed button"=w670:refnum<vi>)
        n242 = Match Pattern(string=w689, regular expression=",") -> (before substring=w694:string, after substring=w693:string)  [unwired: 1 in, 2 out]
        n243 = call <vilib>:"Build State String with Arguments__JKI_lib_State_Machine.vi"("Arguments (\"\")"=w689, "State"=w690) -> ("State with Arguments"=w688:string)  [unwired: 4 in]
        n244 = Fract/Exp String To Number(string=w693) -> (number=w686:dbl)  [unwired: 3 in, 1 out]
        n245 = call "daq_input.vi"("error in (no error)"=w687, "channel"="LOAD_CALIBRATION") -> ("error out"=w684:errorcluster, "value"=w685:dbl)  [unwired: 8 in]
        n246 = case shown="\"release\"" w694 {
          tunnel: [w704 1.0 ("Data Value to Write") 0.0 ("Data Value to Write")] -> w695
          tunnel: [1.0 ("Data Value to Write") 1.0 ("Data Value to Write") 0.0 ("Data Value to Write")] -> w692
          tunnel: w686 -> [w703 w712 _]
          tunnel: w685 -> [w700 w713 _]
          tunnel: [w702 w714 TRUE] -> w669
          tunnel: ["Private: Winch action >> Off" "Private: Winch action >> Off" "Private: no-op"] -> w680
          tunnel: [w698 w710 w717] -> w671
          tunnel: w674 -> [w697 w710 w717]
          frame "release" {
            # "turn off the winch\nwhen the value\nis reached"
            # "switches the direction\nof the winch if it notices\nthe force going up\nwhen it should have\nbeen going down"
            n247 = Greater Or Equal?(x=w703, y=w700) -> (x >= y?=w702:bool)
            n248 = Greater Or Equal?(x=w700, y=w697) -> (x >= y?=w699:bool)
            n249 = case shown="True" w699 {
              tunnel: [0.0 ("Data Value to Write") 1.0 ("Data Value to Write")] -> w704
              tunnel: [w706 -9999.0 ("value")] -> w698
              tunnel: w697 -> [w706 _]
              frame False {
              }
              frame True {
              }
            }
          }
          frame "pull" {
            # "turn off the winch\nwhen the value\nis reached"
            n250 = Less Or Equal?(x=w712, y=w713) -> (x <= y?=w714:bool)
          }
          frame "off", Default {
          }
        }
        n251 = property class="Bool (strict)"(reference=w670) -> ("Value"=w667:bool)  [unwired: 1 in, 2 out]
        n252 = Bundle By Name(cluster=w673, "winch parameter"=w671) -> (w672:T12)
        n253 = Or(x=w669, y=w667) -> (x .or. y?=w668:bool)
        n254 = call "daq_output.vi"("error in (no error)"=w684, "value"=w695, "channel"="ACT_WINCH_DIR") -> ("error out"=w683:errorcluster)  [unwired: 8 in]
        n255 = Select(t=w680, s=w668, f=w688) -> (s? t:f=w676:string)
        n256 = Wait (ms)(milliseconds to wait=u32 50) -> ()  [unwired: 1 out]
        n257 = call "daq_output.vi"("error in (no error)"=w683, "value"=w692, "channel"="ACT_WINCH_ON") -> ("error out"=w682:errorcluster)  [unwired: 8 in]
        n258 = call <vilib>:"Add State(s) to Queue__JKI_lib_State_Machine.vi"("State(s) in Front (\"\")"=w676, "State(s) in (\"\")"=w675) -> ("States Out"=w696:string)  [unwired: 13 in]
      }
      frame "Wait for OX Tank Pressure" {
        # "perform the actual function"
        # "check for negative PSI values or non-numerical arguments"
        # "dummy"
        # "Public function performs setup before running \"Private: Wait for OX Tank Pressure\""
        n259 = Fract/Exp String To Number(string=w725, default (0 dbl)=-1.0 ("default (0 DBL)")) -> (number=w727:dbl)  [unwired: 2 in, 1 out]
        n260 = Less Than 0?(x=w727) -> (x < 0?=w729:bool)
        n261 = case shown="True" w729 {
          tunnel: [w739 w745] -> w730
          tunnel: w732 -> [w737 _]
          tunnel: w731 -> [w738 w745]
          frame True {
            w743 = 42 items=["No error", "Argument error", "Memory is full", "Out of zone", "End of file", "File already open", "Generic file I/O error", "File not found", "File permission error", "Disk is full", "Duplicate path", "Too many files open", "System feature not enabled", "Resource file not found", "Cannot add resource", "Resource not found", "Image not found", "Image memory error", "Pen does not exist", "Config type invalid", "Config token not found", "Config parse error", "Config memory error", "Bad external code format", "Bad external code offset", "External code not present", "Null window", "Destroy window error", "Null menu", "Print aborted", "Bad print record", "Print driver error", "Windows error during printing", "Memory error during printing", "Print dialog error", "Generic print error", "Invalid device refnum", "Device not found", "Device parameter error", "Device unit error", "Cannot open device", "Device call aborted", "Generic error", "Cancelled by user", "Object ID too low", "Object ID too high", "Object not in heap", "Unknown heap", "Unknown object (invalid DefProc)", "Unknown object (DefProc not in table)", "Message out of range", "Invalid (null) method", "Unknown message", "Manager call not supported", "Bad address", "Network operation in progress", "Network operation timed out", "Connection is busy", "Network attribute not supported", "Network error", "Address in use", "System out of memory", "Connection aborted", "Connection refused", "Not connected", "Already connected", "Connection closed", "Initialization error (interapplication manager)", "Bad occurrence", "Wait on unbound occurrence handler", "Occurrence queue overflow", "Datalog type conflict", "Unused", "Unrecognized type (interapplication manager)", "Memory corrupt", "Failed to make temporary DLL", "Old CIN version", "Drag socket not found", "Failed to load drop-object", "Failed to register OLE object", "Failed to release OLE object", "Format specifier type mismatch", "Unknown format specifier", "Too few format specifiers", "Too many format specifiers", "Scan failed", "Newer CIN version", "Error converting to variant", "Runtime menu error", "Password tampered", "Variant attribute not found", "Incompatible variant data type", "Event data is not available", "Event Store is not present", "Occurrence is not found", "Event Queue is not created", "Event info is not available", "Refnum passed is NULL", "Error retrieving Class GUID", "Error retrieving CoClass GUID", "Error retrieving TypeLib GUID.", "Bad built application magic bytes.", "Specific driver is different from the specific driver associated with the Logical Name.", "There is no session opened to the class driver.", "Max Error", "MAX - Error with config objects", "MAX - Error loading configuration", "MAX - Group not supported"]
            n262 = Format Into String(format string="Software Exception: Invalid PSI value argument passed to \"%s\"" ("message"), error in=w738, w737) -> (resulting string=w742:string, error out=w741:errorcluster)  [unwired: 1 in]
            n263 = call <vilib>:"Error Cluster From Error Code.vi"("show call chain? (False)"=TRUE, "error in (no error)"=w741, "error message (\"\")"=w742, "error code (0)"=w743) -> ("error out"=w739:errorcluster)  [unwired: 5 in]
          }
          frame False {
          }
        }
        n264 = call <vilib>:"Build State String with Arguments__JKI_lib_State_Machine.vi"("Arguments (\"\")"=w725, "State"="Private: Wait for OX Tank Pressure") -> ("State with Arguments"=w722:string)  [unwired: 4 in]
        n265 = Concatenate Strings("UI: Proceed Button >> Enable", "\n", w722) -> (w728:string)
        n266 = call <vilib>:"Add State(s) to Queue__JKI_lib_State_Machine.vi"("State(s) in Front (\"\")"=w728, "State(s) in (\"\")"=w734) -> ("States Out"=w736:string)  [unwired: 13 in]
      }
      frame "Private: Wait for OX Tank Pressure" {
        # "Poll the pressure reading in the PSI_TANK_OX until we reach the correct value"
        n267 = call <vilib>:"Build State String with Arguments__JKI_lib_State_Machine.vi"("Arguments (\"\")"=w748, "State"=w762) -> ("State with Arguments"=w758:string)  [unwired: 4 in]
        n268 = Fract/Exp String To Number(string=w748) -> (number=w749:dbl)  [unwired: 3 in, 1 out]
        n269 = Unbundle By Name(w747) -> ("proceed button"=w746:refnum<vi>)
        n270 = property on="Property Node" class="Bool (strict)"(reference=w746, error in=w761) -> (error out=w751:errorcluster, "Value"=w756:bool)  [unwired: 1 out]
        n271 = Wait (ms)(milliseconds to wait=u32 50) -> ()  [unwired: 1 out]
        n272 = call "daq_input.vi"("error in (no error)"=w751, "channel"="PSI_TANK_OX") -> ("error out"=w759:errorcluster, "value"=w755:dbl)  [unwired: 8 in]
        n273 = Greater?(x=w755, y=w749) -> (0:w757:bool)
        n274 = Or(x=w756, y=w757) -> (x .or. y?=w754:bool)
        n275 = Select(t="UI: Proceed Button >> Disable", s=w754, f=w758) -> (s? t:f=w760:string)
        n276 = call <vilib>:"Add State(s) to Queue__JKI_lib_State_Machine.vi"("State(s) in Front (\"\")"=w760, "State(s) in (\"\")"=w763) -> ("States Out"=w764:string)  [unwired: 13 in]
      }
      frame "Start Countdown" {
        # "Set up at countdown indicator and sounds to run asynchronously"
        n277 = Unbundle By Name(w765) -> ("mode"=w766:enum16{"online", "demo", "compile"})
        n278 = case shown="\"online\", \"demo\", Default" w766 {
          tunnel: w770 -> [w772 w778]
          tunnel: [w772 w777] -> w769
          tunnel: w767 -> [_ w775]
          frame "compile" {
          }
          frame "online", "demo", Default {
            w779 = 128  # call and forget
            # "Asyncronous call to countdown subvi.\nState will move on without waiting for results."
            n279 = vi-ref "countdown.vi"() -> (w773:refnum<vi>)
            n280 = property class="VI"(reference=w773, error in=w778) -> (error out=w785:errorcluster, "Name"=w784:string)  [unwired: 1 out]
            n281 = invoke on="Countdown Sub Panel - Auto Sequence" class="SubPnl" method="Insert VI"("VI Ref"=w773) -> ()  [unwired: 3 in, 4 out]
            n282 = Fract/Exp String To Number(string=w775, default (0 dbl)=-1.0 ("default (0 DBL)")) -> (number=w774:dbl)  [unwired: 2 in, 1 out]
            n283 = Open VI Reference(type specifier VI Refnum (for type only)=refnum<vi> refnum, vi path=w784, options=w779, error in (no error)=w785) -> (vi reference=w781:refnum<vi>, error out=w782:errorcluster)  [unwired: 2 in]
            n284 = call-by-ref "Start Asynchronous Call"(reference=w781, error in=w782, "countdown time\n(sec)"=w774) -> (reference out=w786:refnum<vi>, error out=w783:errorcluster)  [unwired: 11 in]
            n285 = Close Reference(reference=w786, error in (no error)=w783) -> (error out=w777:errorcluster)
          }
        }
        n286 = call <vilib>:"Add State(s) to Queue__JKI_lib_State_Machine.vi"("State(s) in (\"\")"=w768) -> ("States Out"=w771:string)  [unwired: 14 in]
      }
      frame "---------- General Commands ----------" {
        # "Template Separator\n(You can make a copy of, or modify, this frame)"
        n287 = call <vilib>:"Add State(s) to Queue__JKI_lib_State_Machine.vi"("State(s) in (\"\")"=w790) -> ("States Out"=w789:string)  [unwired: 14 in]
      }
      frame "Status" {
        # "Continues to next state\n(no operation)"
        n288 = call <vilib>:"Add State(s) to Queue__JKI_lib_State_Machine.vi"("State(s) in (\"\")"=w795) -> ("States Out"=w794:string)  [unwired: 14 in]
        "STATUS" <- w791
      }
      frame "Wait" {
        # "Set starting time for the \"Private: Wait\" function"
        # "check for negative seconds values or non-numerical arguments"
        # "perform the actual function"
        # "Public function performs setup before running \"Private: Wait\""
        n289 = Fract/Exp String To Number(string=w803, default (0 dbl)=-1.0 ("default (0 DBL)")) -> (number=w802:dbl)  [unwired: 2 in, 1 out]
        n290 = Less Than 0?(x=w802) -> (x < 0?=w808:bool)
        n291 = Equal To 0?(x=w802) -> (x = 0?=w796:bool)
        n292 = case shown="True" w808 {
          tunnel: [w819 w822] -> w810
          tunnel: w809 -> [w816 w822]
          tunnel: w803 -> [w817 _]
          frame True {
            w821 = 42 items=["No error", "Argument error", "Memory is full", "Out of zone", "End of file", "File already open", "Generic file I/O error", "File not found", "File permission error", "Disk is full", "Duplicate path", "Too many files open", "System feature not enabled", "Resource file not found", "Cannot add resource", "Resource not found", "Image not found", "Image memory error", "Pen does not exist", "Config type invalid", "Config token not found", "Config parse error", "Config memory error", "Bad external code format", "Bad external code offset", "External code not present", "Null window", "Destroy window error", "Null menu", "Print aborted", "Bad print record", "Print driver error", "Windows error during printing", "Memory error during printing", "Print dialog error", "Generic print error", "Invalid device refnum", "Device not found", "Device parameter error", "Device unit error", "Cannot open device", "Device call aborted", "Generic error", "Cancelled by user", "Object ID too low", "Object ID too high", "Object not in heap", "Unknown heap", "Unknown object (invalid DefProc)", "Unknown object (DefProc not in table)", "Message out of range", "Invalid (null) method", "Unknown message", "Manager call not supported", "Bad address", "Network operation in progress", "Network operation timed out", "Connection is busy", "Network attribute not supported", "Network error", "Address in use", "System out of memory", "Connection aborted", "Connection refused", "Not connected", "Already connected", "Connection closed", "Initialization error (interapplication manager)", "Bad occurrence", "Wait on unbound occurrence handler", "Occurrence queue overflow", "Datalog type conflict", "Unused", "Unrecognized type (interapplication manager)", "Memory corrupt", "Failed to make temporary DLL", "Old CIN version", "Drag socket not found", "Failed to load drop-object", "Failed to register OLE object", "Failed to release OLE object", "Format specifier type mismatch", "Unknown format specifier", "Too few format specifiers", "Too many format specifiers", "Scan failed", "Newer CIN version", "Error converting to variant", "Runtime menu error", "Password tampered", "Variant attribute not found", "Incompatible variant data type", "Event data is not available", "Event Store is not present", "Occurrence is not found", "Event Queue is not created", "Event info is not available", "Refnum passed is NULL", "Error retrieving Class GUID", "Error retrieving CoClass GUID", "Error retrieving TypeLib GUID.", "Bad built application magic bytes.", "Specific driver is different from the specific driver associated with the Logical Name.", "There is no session opened to the class driver.", "Max Error", "MAX - Error with config objects", "MAX - Error loading configuration", "MAX - Group not supported"]
            n293 = Format Into String(format string="Software Exception: Invalid seconds value argument \"%s\" passed to \"Wait\"" ("message"), error in=w816, w817) -> (resulting string=w814:string, error out=w815:errorcluster)  [unwired: 1 in]
            n294 = call <vilib>:"Error Cluster From Error Code.vi"("show call chain? (False)"=TRUE, "error in (no error)"=w815, "error message (\"\")"=w814, "error code (0)"=w821) -> ("error out"=w819:errorcluster)  [unwired: 5 in]
          }
          frame False {
          }
        }
        n295 = call <vilib>:"Build State String with Arguments__JKI_lib_State_Machine.vi"("Arguments (\"\")"=w803, "State"="Private: Wait") -> ("State with Arguments"=w799:string)  [unwired: 4 in]
        n296 = Get Date/Time In Seconds() -> (seconds since 1Jan1904=w807:timestamp)
        n297 = To Double Precision Float(number=w807) -> (double precision float=w805:dbl)
        n298 = Bundle By Name(cluster=w806, "time1"=w805) -> (w804:T12)
        n299 = Select(t="UI: Proceed Button >> Disable", s=w796, f=w799) -> (s? t:f=w797:string)
        n300 = call <vilib>:"Add State(s) to Queue__JKI_lib_State_Machine.vi"("State(s) in Front (\"\")"="UI: Proceed Button >> Enable", "State(s) in (\"\")"=w797, "State(s) at Back (\"\")"=w801) -> ("States Out"=w813:string)  [unwired: 12 in]
      }
      frame "Private: Wait" {
        # "Wait the number of seconds passed as an argument"
        n301 = Unbundle By Name(w825) -> ("time1"=w824:dbl, "proceed button"=w823:refnum<vi>)
        n302 = Get Date/Time In Seconds() -> (seconds since 1Jan1904=w831:timestamp)
        n303 = To Double Precision Float(number=w831) -> (double precision float=w832:dbl)
        n304 = Fract/Exp String To Number(string=w836) -> (number=w826:dbl)  [unwired: 3 in, 1 out]
        n305 = Subtract(x=w832, y=w824) -> (x-y=w830:dbl)
        n306 = property class="Bool (strict)"(reference=w823) -> ("Value"=w829:bool)  [unwired: 1 in, 2 out]
        n307 = Less Or Equal?(x=w826, y=w830) -> (x <= y?=w828:bool)
        n308 = call <vilib>:"Build State String with Arguments__JKI_lib_State_Machine.vi"("Arguments (\"\")"=w836, "State"=w837) -> ("State with Arguments"=w838:string)  [unwired: 4 in]
        n309 = Or(x=w828, y=w829) -> (x .or. y?=w827:bool)
        n310 = Select(t="UI: Proceed Button >> Disable", s=w827, f=w838) -> (s? t:f=w835:string)
        n311 = call <vilib>:"Add State(s) to Queue__JKI_lib_State_Machine.vi"("State(s) in Front (\"\")"=w835, "State(s) in (\"\")"=w834) -> ("States Out"=w840:string)  [unwired: 13 in]
      }
      frame "Private: Wait for Proceed Button" {
        # "Wait in this state until Proceed button is TRUE\n(required proceed button to be Enabled before this)"
        n312 = Unbundle By Name(w844) -> ("proceed button"=w843:refnum<vi>)
        n313 = property class="Bool (strict)"(reference=w843) -> ("Value"=w842:bool)  [unwired: 1 in, 2 out]
        n314 = call <vilib>:"Build State String with Arguments__JKI_lib_State_Machine.vi"("Arguments (\"\")"=w848, "State"=w849) -> ("State with Arguments"=w850:string)  [unwired: 4 in]
        n315 = Select(t="UI: Proceed Button >> Disable", s=w842, f=w850) -> (s? t:f=w847:string)
        n316 = Wait (ms)(milliseconds to wait=u32 50) -> ()  [unwired: 1 out]
        n317 = call <vilib>:"Add State(s) to Queue__JKI_lib_State_Machine.vi"("State(s) in Front (\"\")"=w847, "State(s) in (\"\")"=w846) -> ("States Out"=w852:string)  [unwired: 13 in]
      }
      frame "Abort Condition" {
        w864 = -989898989.0 ("default (0 DBL)")
        # "check for which version of the abort function to use"
        # "check for non-numerical range"
        # "check for non-existant channel name"
        # "dummy value that\nno one would ever use"
        # "check for negative seconds values or non-numerical arguments"
        # "Set starting time for the \"Private: Abort Condition\" function"
        # "perform the actual function"
        # "Public function performs setup before running \"Private: Abort Condition\""
        n318 = Match Pattern(string=w870, regular expression=",") -> (before substring=w871:string, after substring=w873:string)  [unwired: 1 in, 2 out]
        n319 = Match Pattern(string=w873, regular expression=",") -> (before substring=w859:string, after substring=w876:string)  [unwired: 1 in, 2 out]
        n320 = Match Pattern(string=w876, regular expression=",") -> (before substring=w875:string, after substring=w877:string)  [unwired: 1 in, 2 out]
        n321 = Match Pattern(string=w877, regular expression=",") -> (before substring=w874:string, after substring=w856:string)  [unwired: 1 in, 2 out]
        n322 = case shown="\"never\"" w856 {
          tunnel: [FALSE FALSE TRUE] -> w855
          tunnel: ["UI: Proceed Button >> Enable\nPrivate: Abort if never in range" "UI: Proceed Button >> Enable\nPrivate: Abort if ever in range" "" ("regular expression")] -> w854
          frame "never" {
          }
          frame "ever" {
          }
          frame Default {
          }
        }
        n323 = To Upper Case(1:w859) -> (0:w858:string)
        n324 = Fract/Exp String To Number(string=w874, default (0 dbl)=w864) -> (number=w865:dbl)  [unwired: 2 in, 1 out]
        n325 = Fract/Exp String To Number(string=w871, default (0 dbl)=-1.0 ("default (0 DBL)")) -> (number=w869:dbl)  [unwired: 2 in, 1 out]
        n326 = call "daq_input.vi"("error in (no error)"=w860, "channel"=w858) -> ("error out"=w867:errorcluster)  [unwired: 8 in, 1 out]
        n327 = Fract/Exp String To Number(string=w875, default (0 dbl)=w864) -> (number=w866:dbl)  [unwired: 2 in, 1 out]
        n328 = Less Than 0?(x=w869) -> (x < 0?=w863:bool)
        n329 = Equal?(x=w866, y=w864) -> (x = y?=w862:bool)
        n330 = Equal?(x=w865, y=w864) -> (x = y?=w861:bool)
        n331 = Compound Arithmetic op=OR(w863, w862, w861, w855) -> (w857:bool)
        n332 = case shown="True" w857 {
          tunnel: [w899 w902] -> w886
          tunnel: w867 -> [w896 w902]
          tunnel: w870 -> [w897 _]
          frame True {
            w901 = 42 items=["No error", "Argument error", "Memory is full", "Out of zone", "End of file", "File already open", "Generic file I/O error", "File not found", "File permission error", "Disk is full", "Duplicate path", "Too many files open", "System feature not enabled", "Resource file not found", "Cannot add resource", "Resource not found", "Image not found", "Image memory error", "Pen does not exist", "Config type invalid", "Config token not found", "Config parse error", "Config memory error", "Bad external code format", "Bad external code offset", "External code not present", "Null window", "Destroy window error", "Null menu", "Print aborted", "Bad print record", "Print driver error", "Windows error during printing", "Memory error during printing", "Print dialog error", "Generic print error", "Invalid device refnum", "Device not found", "Device parameter error", "Device unit error", "Cannot open device", "Device call aborted", "Generic error", "Cancelled by user", "Object ID too low", "Object ID too high", "Object not in heap", "Unknown heap", "Unknown object (invalid DefProc)", "Unknown object (DefProc not in table)", "Message out of range", "Invalid (null) method", "Unknown message", "Manager call not supported", "Bad address", "Network operation in progress", "Network operation timed out", "Connection is busy", "Network attribute not supported", "Network error", "Address in use", "System out of memory", "Connection aborted", "Connection refused", "Not connected", "Already connected", "Connection closed", "Initialization error (interapplication manager)", "Bad occurrence", "Wait on unbound occurrence handler", "Occurrence queue overflow", "Datalog type conflict", "Unused", "Unrecognized type (interapplication manager)", "Memory corrupt", "Failed to make temporary DLL", "Old CIN version", "Drag socket not found", "Failed to load drop-object", "Failed to register OLE object", "Failed to release OLE object", "Format specifier type mismatch", "Unknown format specifier", "Too few format specifiers", "Too many format specifiers", "Scan failed", "Newer CIN version", "Error converting to variant", "Runtime menu error", "Password tampered", "Variant attribute not found", "Incompatible variant data type", "Event data is not available", "Event Store is not present", "Occurrence is not found", "Event Queue is not created", "Event info is not available", "Refnum passed is NULL", "Error retrieving Class GUID", "Error retrieving CoClass GUID", "Error retrieving TypeLib GUID.", "Bad built application magic bytes.", "Specific driver is different from the specific driver associated with the Logical Name.", "There is no session opened to the class driver.", "Max Error", "MAX - Error with config objects", "MAX - Error loading configuration", "MAX - Group not supported"]
            n333 = Format Into String(format string="Software Exception: Invalid argument \"%s\" passed to \"Abort Condition\"" ("message"), error in=w896, w897) -> (resulting string=w894:string, error out=w895:errorcluster)  [unwired: 1 in]
            n334 = call <vilib>:"Error Cluster From Error Code.vi"("show call chain? (False)"=TRUE, "error in (no error)"=w895, "error message (\"\")"=w894, "error code (0)"=w901) -> ("error out"=w899:errorcluster)  [unwired: 5 in]
          }
          frame False {
          }
        }
        n335 = call <vilib>:"Build State String with Arguments__JKI_lib_State_Machine.vi"("Arguments (\"\")"=w870, "State"=w854) -> ("State with Arguments"=w853:string)  [unwired: 4 in]
        n336 = Get Date/Time In Seconds() -> (seconds since 1Jan1904=w884:timestamp)
        n337 = To Double Precision Float(number=w884) -> (double precision float=w882:dbl)
        n338 = Bundle By Name(cluster=w883, "time1"=w882) -> (w881:T12)
        n339 = call <vilib>:"Add State(s) to Queue__JKI_lib_State_Machine.vi"("State(s) in Front (\"\")"=w853, "State(s) in (\"\")"=w885) -> ("States Out"=w887:string)  [unwired: 13 in]
      }
      frame "Private: Abort if ever in range" {
        # "channels are always uppercase"
        # "if time elapsed and channel stayed\nwithin range, then continue execution"
        # "keep checking until time has elapsed"
        # "if not, ESTOP and stop execution"
        # "check if channel is reading within given range"
        # "Wait the number of seconds passed as an argument, but ESTOP if a channel went out of range"
        n340 = Match Pattern(string=w916, regular expression=",") -> (before substring=w920:string, after substring=w922:string)  [unwired: 1 in, 2 out]
        n341 = Match Pattern(string=w922, regular expression=",") -> (before substring=w914:string, after substring=w925:string)  [unwired: 1 in, 2 out]
        n342 = Match Pattern(string=w925, regular expression=",") -> (before substring=w924:string, after substring=w926:string)  [unwired: 1 in, 2 out]
        n343 = Match Pattern(string=w926, regular expression=",") -> (before substring=w923:string)  [unwired: 1 in, 3 out]
        n344 = call <vilib>:"Build State String with Arguments__JKI_lib_State_Machine.vi"("Arguments (\"\")"=w916, "State"=w941) -> ("State with Arguments"=w908:string)  [unwired: 4 in]
        n345 = To Upper Case(1:w914) -> (0:w913:string)
        n346 = Fract/Exp String To Number(string=w923) -> (number=w910:dbl)  [unwired: 3 in, 1 out]
        n347 = Fract/Exp String To Number(string=w920) -> (number=w919:dbl)  [unwired: 3 in, 1 out]
        n348 = Fract/Exp String To Number(string=w924) -> (number=w911:dbl)  [unwired: 3 in, 1 out]
        n349 = call "daq_input.vi"("channel"=w913) -> ("value"=w912:dbl)  [unwired: 9 in, 1 out]
        n350 = Unbundle By Name(w932) -> ("time1"=w931:dbl, "proceed button"=w930:refnum<vi>)
        n351 = Concatenate Strings(w908, "\n", w904) -> (w907:string)
        n352 = In Range and Coerce(upper limit=w910, x=w912, lower limit=w911) -> (In Range?=w918:bool)  [unwired: 1 out]
        n353 = Get Date/Time In Seconds() -> (seconds since 1Jan1904=w937:timestamp)
        n354 = Select(t=w907, s=w918, f="DAQ_ARM >> Off\nWait >> 2\nENTRY: Standby") -> (s? t:f=w915:string)
        n355 = To Double Precision Float(number=w937) -> (double precision float=w938:dbl)
        n356 = property class="Bool (strict)"(reference=w930) -> ("Value"=w935:bool)  [unwired: 1 in, 2 out]
        n357 = Subtract(x=w938, y=w931) -> (x-y=w936:dbl)
        n358 = Less Or Equal?(x=w919, y=w936) -> (x <= y?=w934:bool)
        n359 = Or(x=w934, y=w935) -> (x .or. y?=w933:bool)
        n360 = Concatenate Strings("UI: Proceed Button >> Disable" ("t"), "\n", w904) -> (w903:string)
        n361 = Select(t=w903, s=w933, f=w915) -> (s? t:f=w940:string)
        n362 = call <vilib>:"Add State(s) to Queue__JKI_lib_State_Machine.vi"("State(s) in Front (\"\")"=w940) -> ("States Out"=w942:string)  [unwired: 14 in]
      }
      frame "Private: Abort if never in range" {
        # "elapsed time"
        # "if not, then we might abort"
        # "channels are always uppercase"
        # "if time elapsed and channel did not go\nwithin range, then abort"
        # "keep checking until time has elapsed"
        # "if it is, then we might move\n on to the next command"
        # "check if channel is reading within given range"
        # "Wait the number of seconds passed as an argument, but ESTOP if a channel went out of range"
        n363 = Match Pattern(string=w963, regular expression=",") -> (before substring=w965:string, after substring=w967:string)  [unwired: 1 in, 2 out]
        n364 = Match Pattern(string=w967, regular expression=",") -> (before substring=w962:string, after substring=w970:string)  [unwired: 1 in, 2 out]
        n365 = Match Pattern(string=w970, regular expression=",") -> (before substring=w969:string, after substring=w971:string)  [unwired: 1 in, 2 out]
        n366 = Match Pattern(string=w971, regular expression=",") -> (before substring=w968:string)  [unwired: 1 in, 3 out]
        n367 = call <vilib>:"Build State String with Arguments__JKI_lib_State_Machine.vi"("Arguments (\"\")"=w963, "State"=w982) -> ("State with Arguments"=w944:string)  [unwired: 4 in]
        n368 = To Upper Case(1:w962) -> (0:w961:string)
        n369 = Fract/Exp String To Number(string=w968) -> (number=w958:dbl)  [unwired: 3 in, 1 out]
        n370 = Fract/Exp String To Number(string=w965) -> (number=w964:dbl)  [unwired: 3 in, 1 out]
        n371 = Fract/Exp String To Number(string=w969) -> (number=w959:dbl)  [unwired: 3 in, 1 out]
        n372 = call "daq_input.vi"("channel"=w961) -> ("value"=w960:dbl)  [unwired: 9 in, 1 out]
        n373 = Unbundle By Name(w976) -> ("time1"=w975:dbl, "proceed button"=w955:refnum<vi>)
        n374 = In Range and Coerce(upper limit=w958, x=w960, lower limit=w959) -> (In Range?=w953:bool)  [unwired: 1 out]
        n375 = Get Date/Time In Seconds() -> (seconds since 1Jan1904=w978:timestamp)
        n376 = To Double Precision Float(number=w978) -> (double precision float=w979:dbl)
        n377 = property class="Bool (strict)"(reference=w955) -> ("Value"=w952:bool)  [unwired: 1 in, 2 out]
        n378 = Or(x=w953, y=w952) -> (x .or. y?=w954:bool)
        n379 = Subtract(x=w979, y=w975) -> (x-y=w977:dbl)
        n380 = Concatenate Strings("UI: Proceed Button >> Disable" ("t"), "\n", w945) -> (w947:string)
        n381 = Select(t=w947, s=w954, f="DAQ_ARM >> Off\nWait >> 2\nENTRY: Standby") -> (s? t:f=w956:string)
        n382 = Less Or Equal?(x=w964, y=w977) -> (x <= y?=w951:bool)
        n383 = Concatenate Strings(w944, "\n", w945) -> (w943:string)
        n384 = Or(x=w951, y=w952) -> (x .or. y?=w950:bool)
        n385 = Select(t=w956, s=w950, f=w943) -> (s? t:f=w981:string)
        n386 = call <vilib>:"Add State(s) to Queue__JKI_lib_State_Machine.vi"("State(s) in Front (\"\")"=w981) -> ("States Out"=w983:string)  [unwired: 14 in]
      }
      frame "User OK Dialog" {
        # "Enable/Disable the \"Proceed\" UI button\n(the button value affects \"Wait...\" states)"
        n387 = Unbundle By Name(w986) -> ("mode"=w985:enum16{"online", "demo", "compile"})
        n388 = case shown="\"online\", \"demo\", Default" w985 {
          tunnel: w989 -> [_ w998]
          tunnel: w987 -> [w991 w994]
          tunnel: [w991 w992] -> w984
          frame "compile" {
          }
          frame "online", "demo", Default {
            n389 = Two Button Dialog(message=w998, 1:"CANCEL (return to Standby)" ("F button name (\"Cancel\")"), 2:"OK" ("T button name (\"OK\")")) -> (T button?=w993:bool)
            n390 = Select(t=w994, s=w993, f="ENTRY: Standby" ("F button name (\"Cancel\")")) -> (s? t:f=w992:string)
          }
        }
        n391 = call <vilib>:"Add State(s) to Queue__JKI_lib_State_Machine.vi"("State(s) in (\"\")"=w984) -> ("States Out"=w990:string)  [unwired: 14 in]
      }
      frame "---------- End ----------" {
        # "Template Separator\n(You can make a copy of, or modify, this frame)"
        n392 = call <vilib>:"Add State(s) to Queue__JKI_lib_State_Machine.vi"("State(s) in (\"\")"=w1002) -> ("States Out"=w1001:string)  [unwired: 14 in]
      }
      frame "---------- Clean ----------" {
        # "Template Separator\n(You can make a copy of, or modify, this frame)"
        n393 = call <vilib>:"Add State(s) to Queue__JKI_lib_State_Machine.vi"("State(s) in (\"\")"=w1006) -> ("States Out"=w1005:string)  [unwired: 14 in]
      }
      frame "---------- Digital Output ----------" {
        # "Template Separator\n(You can make a copy of, or modify, this frame)"
        n394 = call <vilib>:"Add State(s) to Queue__JKI_lib_State_Machine.vi"("State(s) in (\"\")"=w1010) -> ("States Out"=w1009:string)  [unwired: 14 in]
      }
      frame "Private: Digital Output" {
        # "Set the value on a digital channel\n(Throws an error for invalid argument or invalid channel name)"
        n395 = Unbundle By Name(w1017) -> ("digital logic"=w1016:T11, "channel name"=w1014:string)
        n396 = case shown="\"on/off=1/0\"" w1016 {
          tunnel: w1015 -> [w1023 w1029 w1035 w1041]
          tunnel: [w1022 w1027 w1033 w1039] -> w1013
          tunnel: [w1021 w1028 w1034 w1040] -> w1012
          frame "open/close=1/0", Default {
            n397 = case shown="\"close\"" w1023 {
              tunnel: [0.0 ("Data Value to Write") 1.0 ("Data Value to Write") _] -> w1021
              tunnel: [_ _ TRUE ("show call chain? (False)")] -> w1022
              frame "close" {
              }
              frame "open" {
              }
              frame Default {
              }
            }
          }
          frame "open/close=0/1" {
            n398 = case shown="\"open\"" w1029 {
              tunnel: [0.0 ("Data Value to Write") 1.0 ("Data Value to Write") _] -> w1028
              tunnel: [_ _ TRUE ("show call chain? (False)")] -> w1027
              frame "open" {
              }
              frame "close" {
              }
              frame Default {
              }
            }
          }
          frame "on/off=1/0" {
            n399 = case shown="\"off\"" w1035 {
              tunnel: [0.0 ("Data Value to Write") 1.0 ("Data Value to Write") _] -> w1034
              tunnel: [_ _ TRUE ("show call chain? (False)")] -> w1033
              frame "off" {
              }
              frame "on" {
              }
              frame Default {
              }
            }
          }
          frame "on/off=0/1" {
            n400 = case shown="\"on\"" w1041 {
              tunnel: [0.0 ("Data Value to Write") 1.0 ("Data Value to Write") _] -> w1040
              tunnel: [_ _ TRUE ("show call chain? (False)")] -> w1039
              frame "on" {
              }
              frame "off" {
              }
              frame Default {
              }
            }
          }
        }
        n401 = case shown="False" w1013 {
          tunnel: [w1048 w1052] -> w1019
          tunnel: w1018 -> [w1047 w1051]
          tunnel: w1015 -> [_ w1049]
          tunnel: w1014 -> [w1046 w1050]
          tunnel: w1012 -> [w1045 _]
          frame False {
            n402 = call "daq_output.vi"("error in (no error)"=w1047, "value"=w1045, "channel"=w1046) -> ("error out"=w1048:errorcluster)  [unwired: 8 in]
          }
          frame True {
            w1056 = 42 items=["No error", "Argument error", "Memory is full", "Out of zone", "End of file", "File already open", "Generic file I/O error", "File not found", "File permission error", "Disk is full", "Duplicate path", "Too many files open", "System feature not enabled", "Resource file not found", "Cannot add resource", "Resource not found", "Image not found", "Image memory error", "Pen does not exist", "Config type invalid", "Config token not found", "Config parse error", "Config memory error", "Bad external code format", "Bad external code offset", "External code not present", "Null window", "Destroy window error", "Null menu", "Print aborted", "Bad print record", "Print driver error", "Windows error during printing", "Memory error during printing", "Print dialog error", "Generic print error", "Invalid device refnum", "Device not found", "Device parameter error", "Device unit error", "Cannot open device", "Device call aborted", "Generic error", "Cancelled by user", "Object ID too low", "Object ID too high", "Object not in heap", "Unknown heap", "Unknown object (invalid DefProc)", "Unknown object (DefProc not in table)", "Message out of range", "Invalid (null) method", "Unknown message", "Manager call not supported", "Bad address", "Network operation in progress", "Network operation timed out", "Connection is busy", "Network attribute not supported", "Network error", "Address in use", "System out of memory", "Connection aborted", "Connection refused", "Not connected", "Already connected", "Connection closed", "Initialization error (interapplication manager)", "Bad occurrence", "Wait on unbound occurrence handler", "Occurrence queue overflow", "Datalog type conflict", "Unused", "Unrecognized type (interapplication manager)", "Memory corrupt", "Failed to make temporary DLL", "Old CIN version", "Drag socket not found", "Failed to load drop-object", "Failed to register OLE object", "Failed to release OLE object", "Format specifier type mismatch", "Unknown format specifier", "Too few format specifiers", "Too many format specifiers", "Scan failed", "Newer CIN version", "Error converting to variant", "Runtime menu error", "Password tampered", "Variant attribute not found", "Incompatible variant data type", "Event data is not available", "Event Store is not present", "Occurrence is not found", "Event Queue is not created", "Event info is not available", "Refnum passed is NULL", "Error retrieving Class GUID", "Error retrieving CoClass GUID", "Error retrieving TypeLib GUID.", "Bad built application magic bytes.", "Specific driver is different from the specific driver associated with the Logical Name.", "There is no session opened to the class driver.", "Max Error", "MAX - Error with config objects", "MAX - Error loading configuration", "MAX - Group not supported"]
            n403 = Format Into String(format string="Software Exception: argument \"%s\" is invalid for \"%s\"" ("message"), error in=w1051, w1049, w1050) -> (resulting string=w1055:string, error out=w1054:errorcluster)  [unwired: 1 in]
            n404 = call <vilib>:"Error Cluster From Error Code.vi"("show call chain? (False)"=TRUE, "error in (no error)"=w1054, "error message (\"\")"=w1055, "error code (0)"=w1056) -> ("error out"=w1052:errorcluster)  [unwired: 5 in]
          }
        }
        n405 = call <vilib>:"Add State(s) to Queue__JKI_lib_State_Machine.vi"("State(s) in (\"\")"=w1011) -> ("States Out"=w1020:string)  [unwired: 14 in]
      }
      frame "ACT_FILL_FU", "ACT_FILL_OX", "ACT_MAIN_FU", "ACT_MAIN_OX", "ACT_MBV", "ACT_PRESS_FU", "ACT_PRESS_OX", "ACT_PURGE_FU", "ACT_PURGE_OX", "ACT_R13", "ACT_R14", "ACT_R15", "ACT_R16", "ACT_R17", "ACT_R18", "ACT_R19", "ACT_R20" {
        # "name of digital channel (as defined in test.commander)"
        # "define how to interpret the channel data"
        # "set the value of the digital output to the argument"
        # "Set the value of digital output channel to the argument\n(only modify this frame if the behavior of this channel changed) (you may duplicate this frame)"
        n406 = call <vilib>:"Build State String with Arguments__JKI_lib_State_Machine.vi"("Arguments (\"\")"=w1063, "State"="Private: Digital Output") -> ("State with Arguments"=w1062:string)  [unwired: 4 in]
        n407 = Bundle By Name(cluster=w1061, "digital logic"=T10."open/close=1/0", "channel name"=w1058) -> (w1060:T12)
        n408 = call <vilib>:"Add State(s) to Queue__JKI_lib_State_Machine.vi"("State(s) in Front (\"\")"=w1062, "State(s) in (\"\")"=w1067) -> ("States Out"=w1066:string)  [unwired: 13 in]
      }
      frame "ACTI_VENT_FU", "ACTI_VENT_OX" {
        # "name of digital channel (as defined in test.commander)"
        # "define how to interpret the channel data"
        # "set the value of the digital output to the argument"
        # "Set the value of digital output channel to the argument\n(only modify this frame if the behavior of this channel changed) (you may duplicate this frame)"
        n409 = call <vilib>:"Build State String with Arguments__JKI_lib_State_Machine.vi"("Arguments (\"\")"=w1073, "State"="Private: Digital Output") -> ("State with Arguments"=w1072:string)  [unwired: 4 in]
        n410 = Bundle By Name(cluster=w1071, "digital logic"=T10."open/close=0/1", "channel name"=w1068) -> (w1070:T12)
        n411 = call <vilib>:"Add State(s) to Queue__JKI_lib_State_Machine.vi"("State(s) in Front (\"\")"=w1072, "State(s) in (\"\")"=w1077) -> ("States Out"=w1076:string)  [unwired: 13 in]
      }
      frame "ACT_EMATCH", "ACT_SIREN", "ACT_WINCH_ON", "DAQ_ARM", "DO_ENGINE_1", "DO_ENGINE_2", "DO_ENGINE_3", "DO_ENGINE_4", "LOG_TRIG_ON" {
        # "name of digital channel (as defined in test.commander)"
        # "define how to interpret the channel data"
        # "set the value of the digital output to the argument"
        # "Set the value of digital output channel to the argument\n(only modify this frame if the behavior of this channel changed) (you may duplicate this frame)"
        n412 = call <vilib>:"Build State String with Arguments__JKI_lib_State_Machine.vi"("Arguments (\"\")"=w1083, "State"="Private: Digital Output") -> ("State with Arguments"=w1082:string)  [unwired: 4 in]
        n413 = Bundle By Name(cluster=w1081, "digital logic"=T10."on/off=1/0", "channel name"=w1078) -> (w1080:T12)
        n414 = call <vilib>:"Add State(s) to Queue__JKI_lib_State_Machine.vi"("State(s) in Front (\"\")"=w1082, "State(s) in (\"\")"=w1087) -> ("States Out"=w1086:string)  [unwired: 13 in]
      }
      frame "---------- Wait on Digital Input ----------" {
        # "Template Separator\n(You can make a copy of, or modify, this frame)"
        n415 = call <vilib>:"Add State(s) to Queue__JKI_lib_State_Machine.vi"("State(s) in (\"\")"=w1091) -> ("States Out"=w1090:string)  [unwired: 14 in]
      }
      frame "Private: Wait on Digital Input" {
        # "put a no-op here so the state machine will move on in the queue"
        # "Wait until digital input matches the argument, or timeout is reached\n(Throws an error for invalid argument or invalid channel name)"
        n416 = Unbundle By Name(w1105) -> ("time1"=w1096:dbl, "timeout"=w1104:dbl, "digital logic"=w1098:T11, "channel name"=w1097:string, "mode"=w1094:enum16{"online", "demo", "compile"})
        n417 = call <vilib>:"Build State String with Arguments__JKI_lib_State_Machine.vi"("Arguments (\"\")"=w1111, "State"=w1114) -> ("State with Arguments"=w1113:string)  [unwired: 4 in]
        n418 = Get Date/Time In Seconds() -> (seconds since 1Jan1904=w1107:timestamp)
        n419 = To Double Precision Float(number=w1107) -> (double precision float=w1106:dbl)
        n420 = Subtract(x=w1106, y=w1096) -> (x-y=w1103:dbl)
        n421 = call "daq_input.vi"("error in (no error)"=w1110, "channel"=w1097) -> ("error out"=w1112:errorcluster, "value"=w1117:dbl)  [unwired: 8 in]
        n422 = Greater Or Equal?(x=w1103, y=w1104) -> (x >= y?=w1093:bool)
        n423 = case shown="\"online\", \"demo\", Default" w1094 {
          tunnel: [w1120 TRUE] -> w1092
          tunnel: w1093 -> [w1120 _]
          frame "online", "demo", Default {
          }
          frame "compile" {
            # "instant timeout"
          }
        }
        n424 = case shown="\"open/close=1/0\", Default" w1098 {
          tunnel: w1117 -> [w1124 w1134 w1142 w1151 w1160]
          tunnel: [w1122 w1133 w1140 w1149 FALSE ("INIT?")] -> w1095
          tunnel: w1111 -> [w1125 w1132 w1143 w1152 _]
          tunnel: [w1123 w1131 w1141 w1150 w1161] -> w1100
          frame "open/close=1/0", Default {
            n425 = case shown="Default" w1125 {
              tunnel: [w1127 w1128 _] -> w1123
              tunnel: w1124 -> [w1126 w1129 _]
              tunnel: [_ _ TRUE ("INIT?")] -> w1122
              frame "close" {
                n426 = Equal To 0?(x=w1126) -> (x = 0?=w1127:bool)
              }
              frame "open" {
                n427 = Not Equal To 0?(x=w1129) -> (x != 0?=w1128:bool)
              }
              frame Default {
              }
            }
          }
          frame "open/close=0/1" {
            n428 = case shown="\"close\"" w1132 {
              tunnel: [w1136 w1137 _] -> w1131
              tunnel: w1134 -> [w1135 w1138 _]
              tunnel: [_ _ TRUE ("INIT?")] -> w1133
              frame "open" {
                n429 = Equal To 0?(x=w1135) -> (x = 0?=w1136:bool)
              }
              frame "close" {
                n430 = Not Equal To 0?(x=w1138) -> (x != 0?=w1137:bool)
              }
              frame Default {
              }
            }
          }
          frame "on/off=1/0" {
            n431 = case shown="\"on\"" w1143 {
              tunnel: [w1145 w1146 _] -> w1141
              tunnel: w1142 -> [w1144 w1147 _]
              tunnel: [_ _ TRUE ("INIT?")] -> w1140
              frame "off" {
                n432 = Equal To 0?(x=w1144) -> (x = 0?=w1145:bool)
              }
              frame "on" {
                n433 = Not Equal To 0?(x=w1147) -> (x != 0?=w1146:bool)
              }
              frame Default {
              }
            }
          }
          frame "on/off=0/1" {
            n434 = case shown="\"off\"" w1152 {
              tunnel: [w1154 w1155 _] -> w1150
              tunnel: w1151 -> [w1153 w1156 _]
              tunnel: [_ _ TRUE ("INIT?")] -> w1149
              frame "on" {
                n435 = Equal To 0?(x=w1153) -> (x = 0?=w1154:bool)
              }
              frame "off" {
                n436 = Not Equal To 0?(x=w1156) -> (x != 0?=w1155:bool)
              }
              frame Default {
              }
            }
          }
          frame "logger_progress" {
            n437 = Not Equal?(x=w1160, y=100.0) -> (x != y?=w1163:bool)
            n438 = Not Equal To 0?(x=w1160) -> (x != 0?=w1162:bool)
            n439 = And(x=w1162, y=w1163) -> (x .and. y?=w1161:bool)
          }
        }
        n440 = Or(x=w1092, y=w1100) -> (x .or. y?=w1108:bool)
        n441 = Not(x=w1100) -> (.not. x?=w1101:bool)
        n442 = And(x=w1092, y=w1101) -> (x .and. y?=w1099:bool)
        n443 = case shown="False" w1095 {
          tunnel: [w1169 w1173] -> w1116
          tunnel: w1112 -> [w1165 w1172]
          tunnel: w1111 -> [w1166 w1171]
          tunnel: w1097 -> [w1167 w1170]
          tunnel: w1099 -> [w1168 _]
          tunnel: w1103 -> [w1164 _]
          frame False {
            # "generate an error if timeout occured"
            n444 = call "fbk_timeout_error.vi"("timeout?"=w1168, "error in (no error)"=w1165, "argument"=w1166, "channel"=w1167, "timeout time"=w1164) -> ("error out"=w1169:errorcluster)  [unwired: 6 in]
          }
          frame True {
            w1177 = 42 items=["No error", "Argument error", "Memory is full", "Out of zone", "End of file", "File already open", "Generic file I/O error", "File not found", "File permission error", "Disk is full", "Duplicate path", "Too many files open", "System feature not enabled", "Resource file not found", "Cannot add resource", "Resource not found", "Image not found", "Image memory error", "Pen does not exist", "Config type invalid", "Config token not found", "Config parse error", "Config memory error", "Bad external code format", "Bad external code offset", "External code not present", "Null window", "Destroy window error", "Null menu", "Print aborted", "Bad print record", "Print driver error", "Windows error during printing", "Memory error during printing", "Print dialog error", "Generic print error", "Invalid device refnum", "Device not found", "Device parameter error", "Device unit error", "Cannot open device", "Device call aborted", "Generic error", "Cancelled by user", "Object ID too low", "Object ID too high", "Object not in heap", "Unknown heap", "Unknown object (invalid DefProc)", "Unknown object (DefProc not in table)", "Message out of range", "Invalid (null) method", "Unknown message", "Manager call not supported", "Bad address", "Network operation in progress", "Network operation timed out", "Connection is busy", "Network attribute not supported", "Network error", "Address in use", "System out of memory", "Connection aborted", "Connection refused", "Not connected", "Already connected", "Connection closed", "Initialization error (interapplication manager)", "Bad occurrence", "Wait on unbound occurrence handler", "Occurrence queue overflow", "Datalog type conflict", "Unused", "Unrecognized type (interapplication manager)", "Memory corrupt", "Failed to make temporary DLL", "Old CIN version", "Drag socket not found", "Failed to load drop-object", "Failed to register OLE object", "Failed to release OLE object", "Format specifier type mismatch", "Unknown format specifier", "Too few format specifiers", "Too many format specifiers", "Scan failed", "Newer CIN version", "Error converting to variant", "Runtime menu error", "Password tampered", "Variant attribute not found", "Incompatible variant data type", "Event data is not available", "Event Store is not present", "Occurrence is not found", "Event Queue is not created", "Event info is not available", "Refnum passed is NULL", "Error retrieving Class GUID", "Error retrieving CoClass GUID", "Error retrieving TypeLib GUID.", "Bad built application magic bytes.", "Specific driver is different from the specific driver associated with the Logical Name.", "There is no session opened to the class driver.", "Max Error", "MAX - Error with config objects", "MAX - Error loading configuration", "MAX - Group not supported"]
            n445 = Format Into String(format string="Software Exception: argument \"%s\" is invalid for \"%s\"." ("message"), error in=w1172, w1171, w1170) -> (resulting string=w1176:string, error out=w1175:errorcluster)  [unwired: 1 in]
            n446 = call <vilib>:"Error Cluster From Error Code.vi"("show call chain? (False)"=TRUE, "error in (no error)"=w1175, "error message (\"\")"=w1176, "error code (0)"=w1177) -> ("error out"=w1173:errorcluster)  [unwired: 5 in]
          }
        }
        n447 = Select(t="Private: no-op", s=w1108, f=w1113) -> (s? t:f=w1115:string)
        n448 = Wait (ms)(milliseconds to wait=u32 50) -> ()  [unwired: 1 out]
        n449 = call <vilib>:"Add State(s) to Queue__JKI_lib_State_Machine.vi"("State(s) in Front (\"\")"=w1115, "State(s) in (\"\")"=w1119) -> ("States Out"=w1118:string)  [unwired: 13 in]
      }
      frame "FBK_FILL_FU", "FBK_FILL_OX", "FBK_L12", "FBK_L13", "FBK_L14", "FBK_L15", "FBK_L16", "FBK_L17", "FBK_L18", "FBK_L19", "FBK_L20", "FBK_MAIN_FU", "FBK_MAIN_OX", "FBK_MBV", "FBK_PRESS_FU", "FBK_PRESS_OX", "FBK_PURGE_FU", "FBK_PURGE_OX", "FBK_VENT_FU", "FBK_VENT_OX" {
        # "argument (open/close/on/off/etc.)"
        # "default timeout"
        # "name of digital channel (as defined in test.commander)"
        # "timeout (maximum time to wait for feedback to match the argument)"
        # "set start time for timeout check"
        # "wait for channel data to match the argument"
        # "define how to interpret the channel data"
        # "Wait for digital input channel to match argument\n(only modify this frame if the behavior of this channel changed) (you may duplicate this frame)"
        n450 = Match Pattern(string=w1183, regular expression=",") -> (before substring=w1180:string, after substring=w1182:string)  [unwired: 1 in, 2 out]
        n451 = Fract/Exp String To Number(string=w1182, default (0 dbl)=5.0 ("default (0 DBL)")) -> (number=w1181:dbl)  [unwired: 2 in, 1 out]
        n452 = Get Date/Time In Seconds() -> (seconds since 1Jan1904=w1190:timestamp)
        n453 = To Double Precision Float(number=w1190) -> (double precision float=w1189:dbl)
        n454 = call <vilib>:"Build State String with Arguments__JKI_lib_State_Machine.vi"("Arguments (\"\")"=w1180, "State"="Private: Wait on Digital Input") -> ("State with Arguments"=w1187:string)  [unwired: 4 in]
        n455 = Bundle By Name(cluster=w1193, "time1"=w1189, "timeout"=w1181, "digital logic"=T11."open/close=1/0", "channel name"=w1186) -> (w1192:T12)
        n456 = call <vilib>:"Add State(s) to Queue__JKI_lib_State_Machine.vi"("State(s) in Front (\"\")"=w1187, "State(s) in (\"\")"=w1188) -> ("States Out"=w1195:string)  [unwired: 13 in]
      }
      frame "ARMED" {
        # "argument (open/close/on/off/etc.)"
        # "default timeout"
        # "name of digital channel (as defined in test.commander)"
        # "timeout (maximum time to wait for feedback to match the argument)"
        # "set start time for timeout check"
        # "wait for channel data to match the argument"
        # "define how to interpret the channel data"
        # "Wait for digital input channel to match argument\n(only modify this frame if the behavior of this channel changed) (you may duplicate this frame)"
        n457 = Match Pattern(string=w1200, regular expression=",") -> (before substring=w1197:string, after substring=w1199:string)  [unwired: 1 in, 2 out]
        n458 = Fract/Exp String To Number(string=w1199, default (0 dbl)=5.0 ("default (0 DBL)")) -> (number=w1198:dbl)  [unwired: 2 in, 1 out]
        n459 = Get Date/Time In Seconds() -> (seconds since 1Jan1904=w1207:timestamp)
        n460 = To Double Precision Float(number=w1207) -> (double precision float=w1206:dbl)
        n461 = call <vilib>:"Build State String with Arguments__JKI_lib_State_Machine.vi"("Arguments (\"\")"=w1197, "State"="Private: Wait on Digital Input") -> ("State with Arguments"=w1204:string)  [unwired: 4 in]
        n462 = Bundle By Name(cluster=w1210, "time1"=w1206, "timeout"=w1198, "digital logic"=T11."on/off=1/0", "channel name"=w1203) -> (w1209:T12)
        n463 = call <vilib>:"Add State(s) to Queue__JKI_lib_State_Machine.vi"("State(s) in Front (\"\")"=w1204, "State(s) in (\"\")"=w1205) -> ("States Out"=w1212:string)  [unwired: 13 in]
      }
      frame "DET_11", "DET_12", "DET_13", "DET_14", "DET_15", "DET_16", "DET_17", "DET_18", "DET_19", "DET_20", "DET_EMATCH", "DET_FILL _OX", "DET_FILL_FU", "DET_MAIN_FU", "DET_MAIN_OX", "DET_PRESS_FU", "DET_PRESS_OX", "DET_PURGE_FU", "DET_PURGE_OX", "DET_VENT_FU", "DET_VENT_OX", "DI_ENGINE_1", "DI_ENGINE_2", "DI_ENGINE_3", "DI_ENGINE_4" {
        # "argument (open/close/on/off/etc.)"
        # "default timeout"
        # "name of digital channel (as defined in test.commander)"
        # "timeout (maximum time to wait for feedback to match the argument)"
        # "set start time for timeout check"
        # "wait for channel data to match the argument"
        # "define how to interpret the channel data"
        # "Wait for digital input channel to match argument\n(only modify this frame if the behavior of this channel changed) (you may duplicate this frame)"
        n464 = Match Pattern(string=w1217, regular expression=",") -> (before substring=w1214:string, after substring=w1216:string)  [unwired: 1 in, 2 out]
        n465 = Fract/Exp String To Number(string=w1216, default (0 dbl)=0.0 ("default (0 DBL)")) -> (number=w1215:dbl)  [unwired: 2 in, 1 out]
        n466 = Get Date/Time In Seconds() -> (seconds since 1Jan1904=w1224:timestamp)
        n467 = To Double Precision Float(number=w1224) -> (double precision float=w1223:dbl)
        n468 = call <vilib>:"Build State String with Arguments__JKI_lib_State_Machine.vi"("Arguments (\"\")"=w1214, "State"="Private: Wait on Digital Input") -> ("State with Arguments"=w1221:string)  [unwired: 4 in]
        n469 = Bundle By Name(cluster=w1227, "time1"=w1223, "timeout"=w1215, "digital logic"=T11."on/off=0/1", "channel name"=w1220) -> (w1226:T12)
        n470 = call <vilib>:"Add State(s) to Queue__JKI_lib_State_Machine.vi"("State(s) in Front (\"\")"=w1221, "State(s) in (\"\")"=w1222) -> ("States Out"=w1229:string)  [unwired: 13 in]
      }
      frame "LOG_TRIG_STATUS" {
        # "argument (open/close/on/off/etc.)"
        # "default timeout"
        # "name of digital channel (as defined in test.commander)"
        # "timeout (maximum time to wait for feedback to match the argument)"
        # "set start time for timeout check"
        # "wait for channel data to match the argument"
        # "define how to interpret the channel data"
        # "Wait for digital input channel to match argument\n(only modify this frame if the behavior of this channel changed) (you may duplicate this frame)"
        n471 = Match Pattern(string=w1234, regular expression=",") -> (before substring=w1231:string, after substring=w1233:string)  [unwired: 1 in, 2 out]
        n472 = Fract/Exp String To Number(string=w1233, default (0 dbl)=5.0 ("default (0 DBL)")) -> (number=w1232:dbl)  [unwired: 2 in, 1 out]
        n473 = Get Date/Time In Seconds() -> (seconds since 1Jan1904=w1241:timestamp)
        n474 = To Double Precision Float(number=w1241) -> (double precision float=w1240:dbl)
        n475 = call <vilib>:"Build State String with Arguments__JKI_lib_State_Machine.vi"("Arguments (\"\")"=w1231, "State"="Private: Wait on Digital Input") -> ("State with Arguments"=w1238:string)  [unwired: 4 in]
        n476 = Bundle By Name(cluster=w1244, "time1"=w1240, "timeout"=w1232, "digital logic"=T11."logger_progress", "channel name"=w1237) -> (w1243:T12)
        n477 = call <vilib>:"Add State(s) to Queue__JKI_lib_State_Machine.vi"("State(s) in Front (\"\")"=w1238, "State(s) in (\"\")"=w1239) -> ("States Out"=w1246:string)  [unwired: 13 in]
      }
      frame "---------- Unused ----------" {
        # "Template Separator\n(You can make a copy of, or modify, this frame)"
        n478 = call <vilib>:"Add State(s) to Queue__JKI_lib_State_Machine.vi"("State(s) in (\"\")"=w1250) -> ("States Out"=w1249:string)  [unwired: 14 in]
      }
      frame "ENTRY: UNUSED1" {
        # "Set up UI and prepare to enter \"Standby\" tab"
        n479 = Wait (ms)(milliseconds to wait=u32 50) -> ()  [unwired: 1 out]
        n480 = call <vilib>:"Add State(s) to Queue__JKI_lib_State_Machine.vi"("State(s) in Front (\"\")"="", "State(s) in (\"\")"=w1256) -> ("States Out"=w1255:string)  [unwired: 13 in]
      }
      frame "Macro: All ACT mimic FBK" {
        # "Initialization Macro\n(This is called once, when the VI starts)"
        n481 = call <vilib>:"Add State(s) to Queue__JKI_lib_State_Machine.vi"("State(s) in Front (\"\")"="Macro: Mimic >> ACT_FILL_FU,FBK_FILL_FU\nMacro: Mimic >> ACT_FILL_OX,FBK_FILL_OX\nMacro: Mimic >> ACT_MAIN_FU,FBK_MAIN_FU\nMacro: Mimic >> ACT_MAIN_OX,FBK_MAIN_OX\nMacro: Mimic >> ACT_MBV,FBK_MBV\nMacro: Mimic >> ACT_PRESS_FU,FBK_PRESS_FU\nMacro: Mimic >> ACT_PRESS_OX,FBK_PRESS_OX\nMacro: Mimic >> ACT_PURGE_FU,FBK_PURGE_FU\nMacro: Mimic >> ACT_PURGE_OX,FBK_PURGE_OX\nMacro: Mimic >> ACTI_VENT_FU,FBK_VENT_FU\nMacro: Mimic >> ACTI_VENT_OX,FBK_VENT_OX\nACT_EMATCH >> Off\nACT_SIREN >> Off\nACT_WINCH_ON >> Off", "State(s) in (\"\")"=w1261) -> ("States Out"=w1260:string)  [unwired: 13 in]
      }
      frame "Macro: Mimic" {
        # "check that the arguments follow\nthe naming convention for actuators\nwith limit switch feedback"
        # "all test.commander variables\nare required to be UPPERCASE"
        # "Initialization Macro\n(This is called once, when the VI starts)"
        n482 = To Upper Case(1:w1263) -> (0:w1262:string)
        n483 = Match Pattern(string=w1262, regular expression=",") -> (before substring=w1272:string, after substring=w1265:string)  [unwired: 1 in, 2 out]
        n484 = Match Pattern(string=w1272, regular expression="^ACT[^_]*") -> (match substring=w1269:string)  [unwired: 1 in, 3 out]
        n485 = Match Pattern(string=w1265, regular expression="^FBK[^_]*") -> (match substring=w1270:string)  [unwired: 1 in, 3 out]
        n486 = Concatenate Strings(w1269, w1270) -> (w1268:string)
        n487 = case shown="\"ACTFBKI\", \"ACTIFBK\"" w1268 {
          tunnel: w1265 -> [_ w1291 w1296]
          tunnel: w1272 -> [_ w1290 w1295]
          tunnel: w1267 -> [w1281 w1285 w1293]
          tunnel: [w1280 w1284 w1294] -> w1266
          tunnel: w1262 -> [w1279 _ _]
          frame Default {
            w1283 = 42 items=["No error", "Argument error", "Memory is full", "Out of zone", "End of file", "File already open", "Generic file I/O error", "File not found", "File permission error", "Disk is full", "Duplicate path", "Too many files open", "System feature not enabled", "Resource file not found", "Cannot add resource", "Resource not found", "Image not found", "Image memory error", "Pen does not exist", "Config type invalid", "Config token not found", "Config parse error", "Config memory error", "Bad external code format", "Bad external code offset", "External code not present", "Null window", "Destroy window error", "Null menu", "Print aborted", "Bad print record", "Print driver error", "Windows error during printing", "Memory error during printing", "Print dialog error", "Generic print error", "Invalid device refnum", "Device not found", "Device parameter error", "Device unit error", "Cannot open device", "Device call aborted", "Generic error", "Cancelled by user", "Object ID too low", "Object ID too high", "Object not in heap", "Unknown heap", "Unknown object (invalid DefProc)", "Unknown object (DefProc not in table)", "Message out of range", "Invalid (null) method", "Unknown message", "Manager call not supported", "Bad address", "Network operation in progress", "Network operation timed out", "Connection is busy", "Network attribute not supported", "Network error", "Address in use", "System out of memory", "Connection aborted", "Connection refused", "Not connected", "Already connected", "Connection closed", "Initialization error (interapplication manager)", "Bad occurrence", "Wait on unbound occurrence handler", "Occurrence queue overflow", "Datalog type conflict", "Unused", "Unrecognized type (interapplication manager)", "Memory corrupt", "Failed to make temporary DLL", "Old CIN version", "Drag socket not found", "Failed to load drop-object", "Failed to register OLE object", "Failed to release OLE object", "Format specifier type mismatch", "Unknown format specifier", "Too few format specifiers", "Too many format specifiers", "Scan failed", "Newer CIN version", "Error converting to variant", "Runtime menu error", "Password tampered", "Variant attribute not found", "Incompatible variant data type", "Event data is not available", "Event Store is not present", "Occurrence is not found", "Event Queue is not created", "Event info is not available", "Refnum passed is NULL", "Error retrieving Class GUID", "Error retrieving CoClass GUID", "Error retrieving TypeLib GUID.", "Bad built application magic bytes.", "Specific driver is different from the specific driver associated with the Logical Name.", "There is no session opened to the class driver.", "Max Error", "MAX - Error with config objects", "MAX - Error loading configuration", "MAX - Group not supported"]
            n488 = Format Into String(format string="Software Exception: \"Macro: Mimic\" was provided with invalid argument \"%s\"" ("message"), w1279) -> (resulting string=w1277:string)  [unwired: 2 in, 1 out]
            n489 = call <vilib>:"Error Cluster From Error Code.vi"("show call chain? (False)"=TRUE, "error in (no error)"=w1281, "error message (\"\")"=w1277, "error code (0)"=w1283) -> ("error out"=w1280:errorcluster)  [unwired: 5 in]
          }
          frame "ACTFBKI", "ACTIFBK" {
            # "Either ACT or FBK has inverted logic (but not both)"
            n490 = call "daq_input.vi"("error in (no error)"=w1285, "channel"=w1291) -> ("error out"=w1286:errorcluster, "value"=w1289:dbl)  [unwired: 8 in]
            n491 = Equal To 0?(x=w1289) -> (x = 0?=w1288:bool)
            n492 = Boolean To (0,1)(Boolean=w1288) -> (0, 1=w1287:i16)
            n493 = call "daq_output.vi"("error in (no error)"=w1286, "value"=w1287, "channel"=w1290) -> ("error out"=w1284:errorcluster)  [unwired: 8 in]
          }
          frame "ACTFBK", "ACTIFBKI" {
            # "normal logic (or double inverted logic)"
            n494 = call "daq_input.vi"("error in (no error)"=w1293, "channel"=w1296) -> ("error out"=w1292:errorcluster, "value"=w1297:dbl)  [unwired: 8 in]
            n495 = call "daq_output.vi"("error in (no error)"=w1292, "value"=w1297, "channel"=w1295) -> ("error out"=w1294:errorcluster)  [unwired: 8 in]
          }
        }
        n496 = call <vilib>:"Add State(s) to Queue__JKI_lib_State_Machine.vi"("State(s) in Front (\"\")"=w1264) -> ("States Out"=w1276:string)  [unwired: 14 in]
      }
    }
  }
  "error out" <- w5
  n497 = for {
    tunnel: w9 -> [w1304] mode=indexing
    tunnel: [w1302] -> w7 mode=indexing
    n498 = Unbundle(w1304) -> (w1298:string, "current time"=w1303:timestamp)
    n499 = call <vilib>:"Space Constant.vi"() -> ("String"=w1300:string)
    n500 = Get Date/Time String(seconds (now)=w1303, want seconds? (F)=TRUE) -> (time string=w1299:string)  [unwired: 1 in, 1 out]
    n501 = Concatenate Strings(w1299, w1300, w1298) -> (w1302:string)
  }
  n502 = call <vilib>:"Application Directory.vi"() -> ("Application Directory"=w2:path)
  n503 = Build Path(base path=w2, name or relative path="log.txt") -> (appended path=w1:path)
  n504 = Write to Text File(file (use dialog)=w1, text=w7) -> ()  [unwired: 2 in, 3 out]
